vi "Main Comic Manager.vi"() -> ()   [LabVIEW 2024]
uses:
  <vilib>/sklein/WebView2/Webview2 Control/WebView2 Control.xctl
  definitions/volume.type--enum.ctl
  definitions/local_volume.ctl
  definitions/local_issue.ctl
  definitions/comicvine_issue.generic_credit.ctl
  definitions/comicvine_issue.associated_image.ctl
  definitions/comicvine_issue.person_credit.ctl
  <vilib>/addons/_JKI Toolkits/State Machine/_JKI_lib_State_Machine.llb/Select State(s)_err__jki_lib_state_machine.vi
  <vilib>/addons/_JKI Toolkits/State Machine/_JKI_lib_State_Machine.llb/Periodic Trigger__ogtk__JKI-SM__jki_lib_state_machine.vi
  <userlib>/_OpenG.lib/array/array.llb/Remove Duplicates from 1D Array (Variant)__ogtk.vi
  <userlib>/_OpenG.lib/file/file.llb/Strip Path Extension - String__ogtk.vi
  <userlib>/_OpenG.lib/file/file.llb/openg_file.lvlib
  <vilib>/addons/_JKI.lib/Serialization/JSON/JKI JSON Serialization.lvlib
  <userlib>/_OpenG.lib/array/array.llb/openg_array.lvlib
panel:
  in  "delete issue":bool caption="delete current"
  in  "use rel date":bool caption="delete current"
  out "issue chart":picture
  in  "fix dates":bool caption="delete current"
  out "dup issues":i32[](array[numeric])
  out "Unique Dates":bool
  in  "delete volume":bool caption="delete current"
  out "URL":string
  in  "refresh listings":bool
  in  "commit volume type":bool
  in  "volume type":T1 caption="Enum"
  out "last updated":string
  in  "Volume":i32 caption="Numeric"
  in  "issue detail tab control":enum32{"Details", "Cover", "Lists"}(tab)
  out "Rel Date":timestamp format="%<%x>T"
  out "Issue ID":i32 caption="Numeric"
  out "Issue Title":string
  in  "Cover Date":timestamp format="%<%x>T"
  out "Issue Number":string
  in  "issue description":string(xcontrol)
  in  "issue cover":string(xcontrol)
  out "Characters":string[](array[string])
  out "Teams":string[](array[string])
  out "StoryArcs":string[](array[string])
  out "Creators":string[](array[string])
  out "Concepts":string[](array[string])
  in  "sort volume":bool
  in  "to top":bool
  in  "move down":bool
  in  "move up":bool
  in  "issues":i32(listbox)
  out "Start Year":i32 caption="Numeric"
  out "issue count":i32 caption="Numeric"
  out "Sortable Title":string
  in  "Title":string
  in  "volume description":string(xcontrol)
  in  "volumes":i32(listbox)
  in  "Folder":i32(listbox)
  in  "Exit":bool
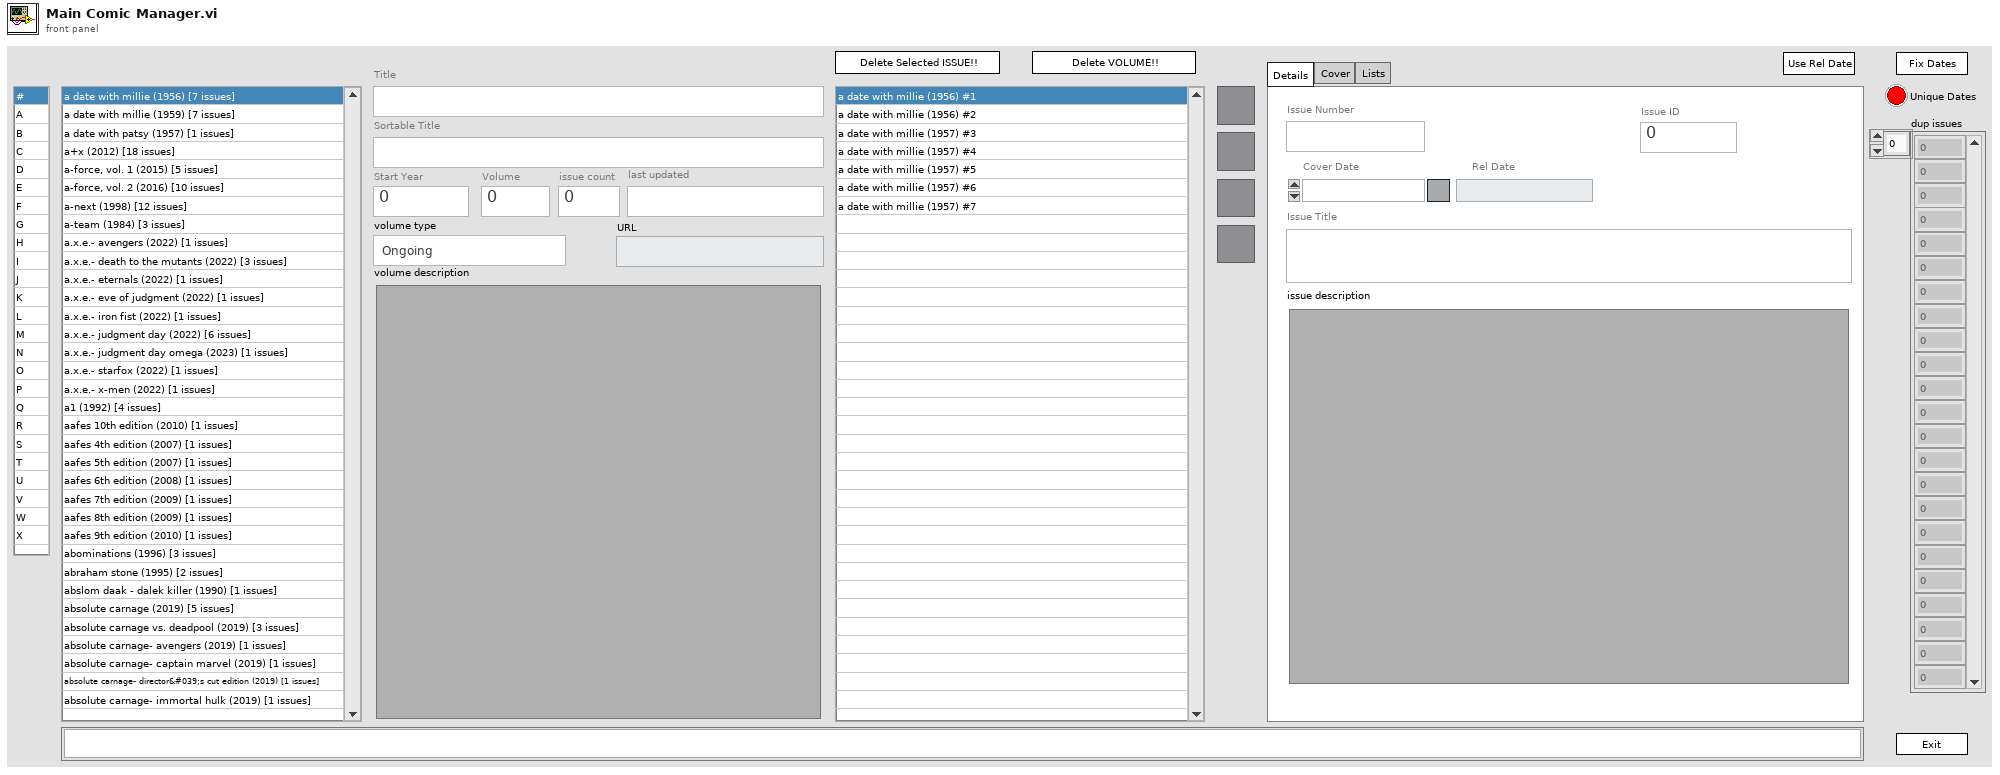
[diagram p1: front panel]
types:
  T1 = typedef "volume.type--enum.ctl" = enum16{"Ongoing", "Limited Series", "Annual", "One Shot", "Reprint/Document", "Star Comics", "Epic Comics"}
  T2 = enum32{"Invalid", "Standard", "Closed", "Hidden", "Minimized", "Maximized"}
  T3 = enum32{"invalid app kind", "Development System", "Run Time System", "Student Edition", "Embedded LabVIEW", "Evaluation", "Custom"}
  T4 = typedef "local_issue.ctl" = cluster{"cover_date":timestamp, "id":i32, "cv_id":string, "name":string, "sortable_name":string, "issue_number":string, "deck":string, "description":string, "volume":T5, "store_date":timestamp, "date_last_updated":timestamp, "site_detail_url":string, "cover_url":string, "associated_images":T6[], "characters":T5[], "concepts":T5[], "creators":T7[], "storyArcs":T5[], "teams":T5[]}
  T5 = typedef "comicvine_issue.generic_credit.ctl" = cluster{"id":i32, "name":string}
  T6 = typedef "comicvine_issue.associated_image.ctl" = cluster{"original_url":string, "id":i32}
  T7 = typedef "comicvine_issue.person_credit.ctl" = cluster{"id":i32, "name":string, "role":string}
  T8 = typedef "local_volume.ctl" = cluster{"id":i32, "name":string, "sortable_name":string, "aliases":string[], "description":string, "site_detail_url":string, "count_of_issues":i32, "start_year":i32, "publisher_id":i32, "issue_ids":i32[], "date_last_updated":timestamp, "volume":i32, "cv_id":string, "volume type":T1}
  T9 = cluster{"Core":cluster{"Current VI Reference":refnum<vi>, "Close Panel on Exit?":bool}, "cv_vols":path[], "vol_filter_map":map{i32, cluster{"name":string, "path":path}[]}, "current_vol_array":cluster{"name":string, "path":path}[], "volume":T8, "issues":T4[], "root paths":cluster{"cv_volumes":path, "cv_issues":path}, "dup issues":i32[]}
  T10 = cluster{"Current VI Reference":refnum<vi>, "Close Panel on Exit?":bool}
  T11 = typedef "WebView2 Control.xctl/Events.ctl" = cluster{"Navigation Complete Event":refnum<user-event>, "Source Changed Event":refnum<user-event>, "Document Title Changed Event":refnum<user-event>, "Status Bar Text Changed":refnum<user-event>, "Web Message Received":refnum<user-event>, "Window Close Requested":refnum<user-event>, "DOM Loaded":refnum<user-event>, "Navigation Started Event":refnum<user-event>}
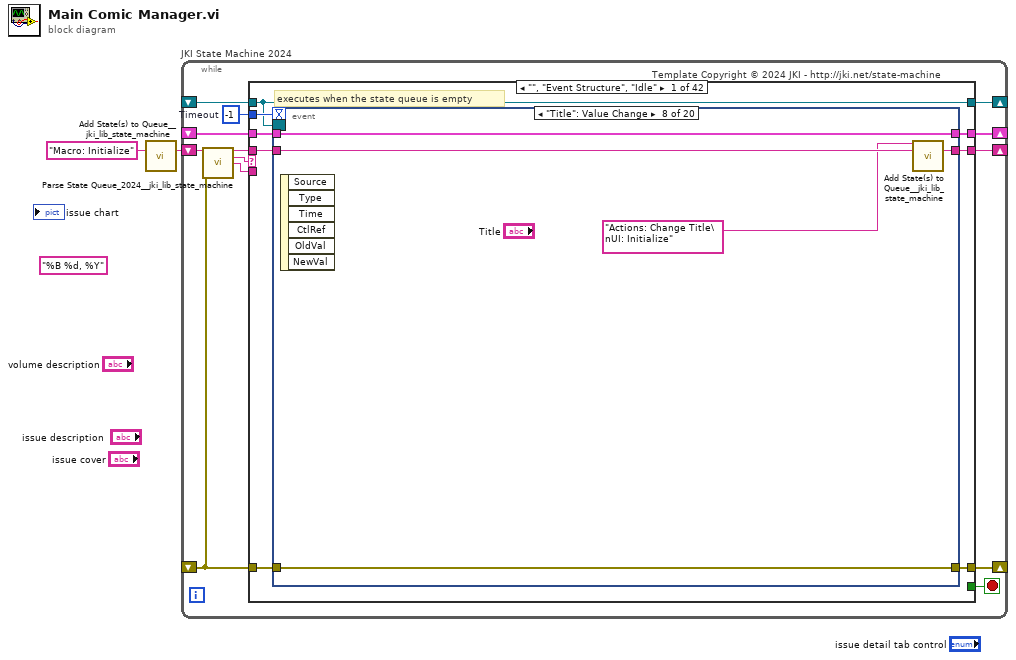
[diagram p0: block diagram]
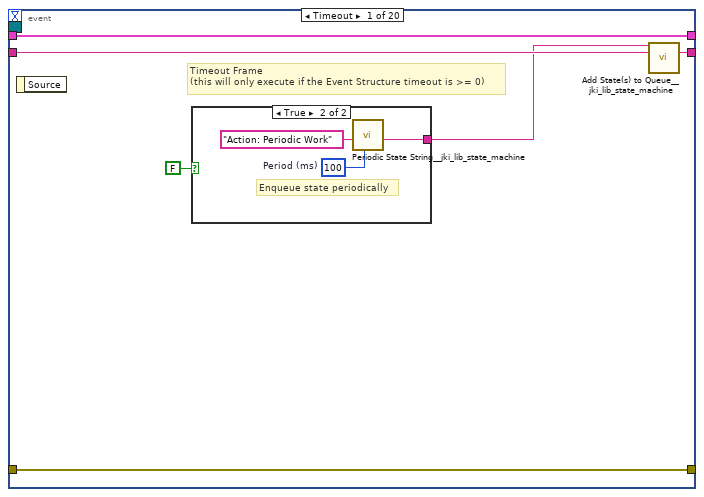
[diagram p2: hidden frame]
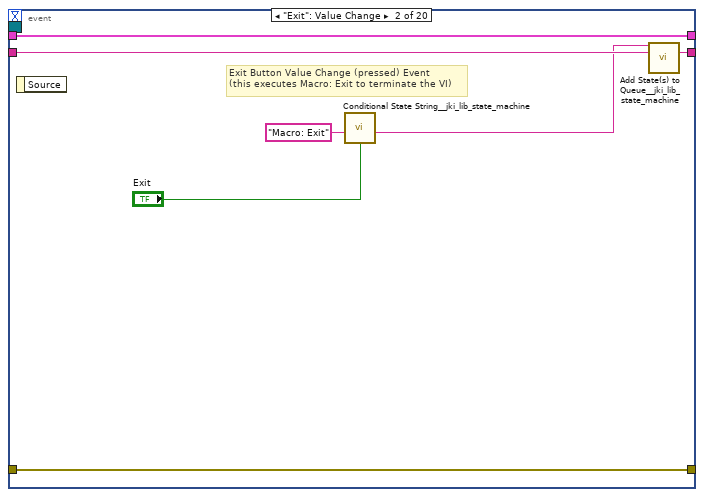
[diagram p4: hidden frame]
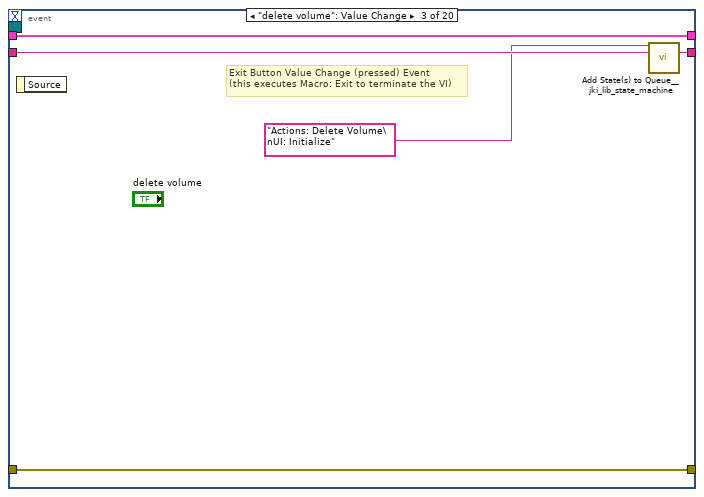
[diagram p5: hidden frame]
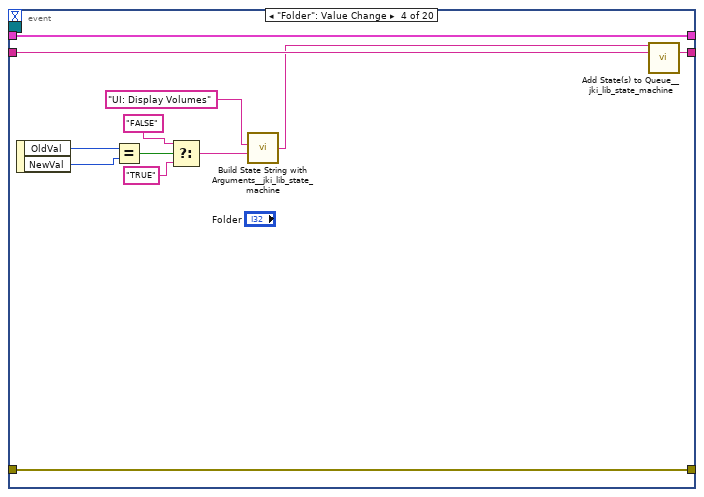
[diagram p6: hidden frame]
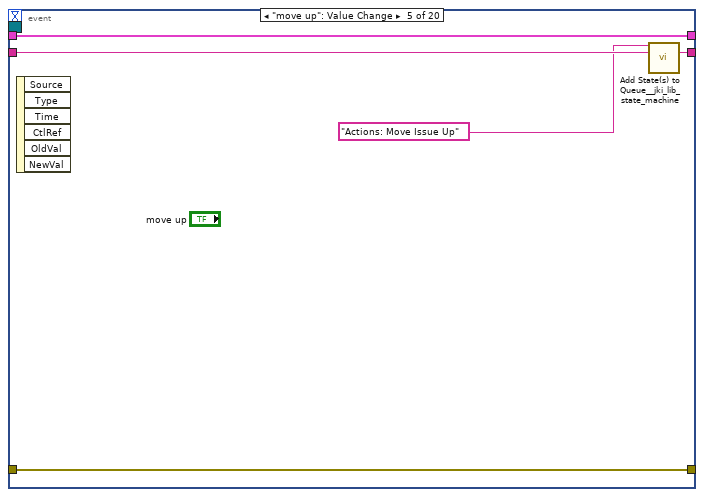
[diagram p7: hidden frame]
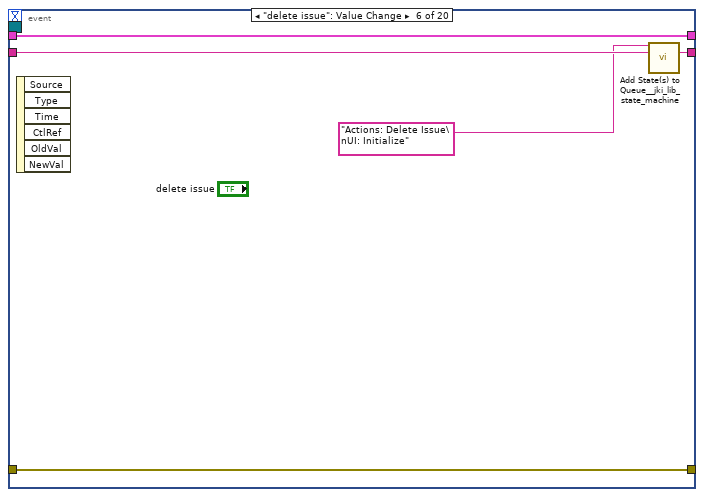
[diagram p8: hidden frame]
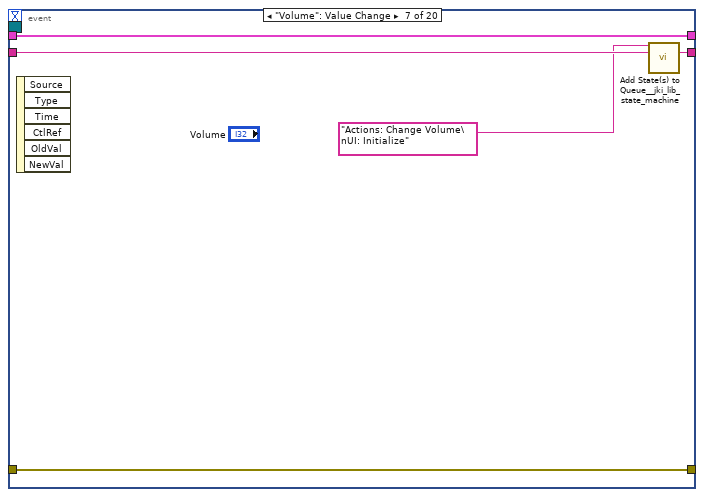
[diagram p9: hidden frame]
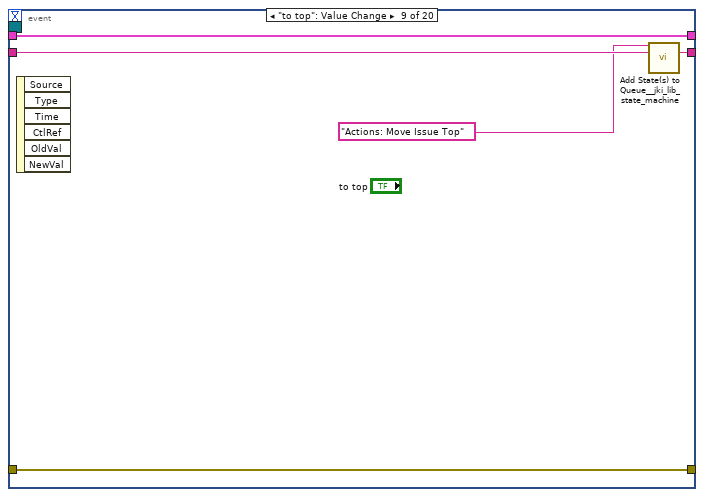
[diagram p10: hidden frame]
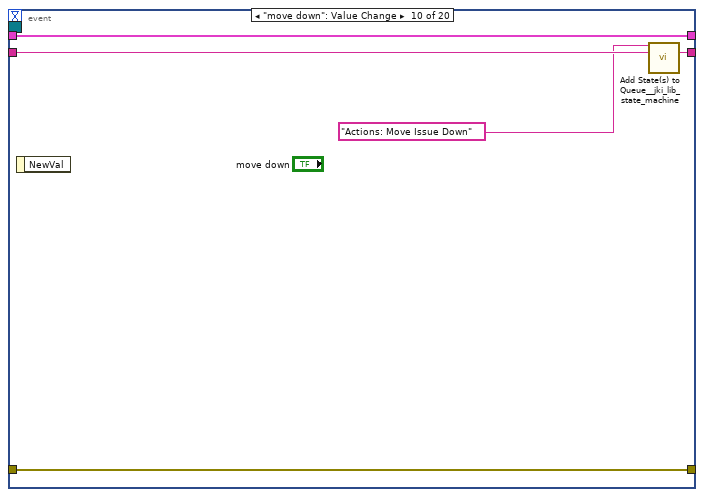
[diagram p11: hidden frame]
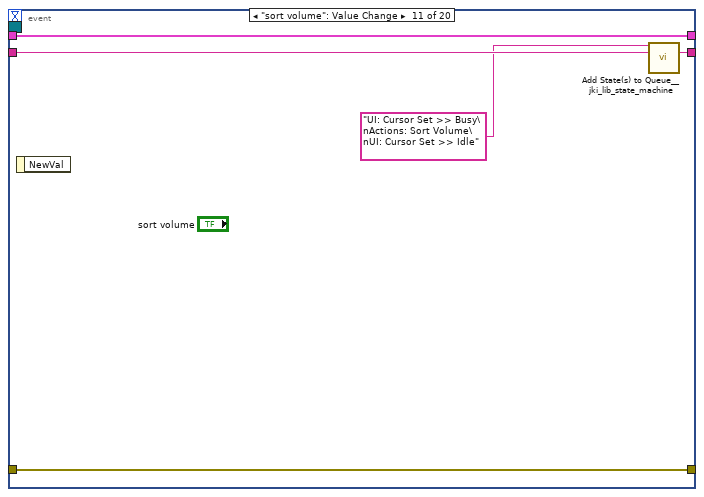
[diagram p12: hidden frame]
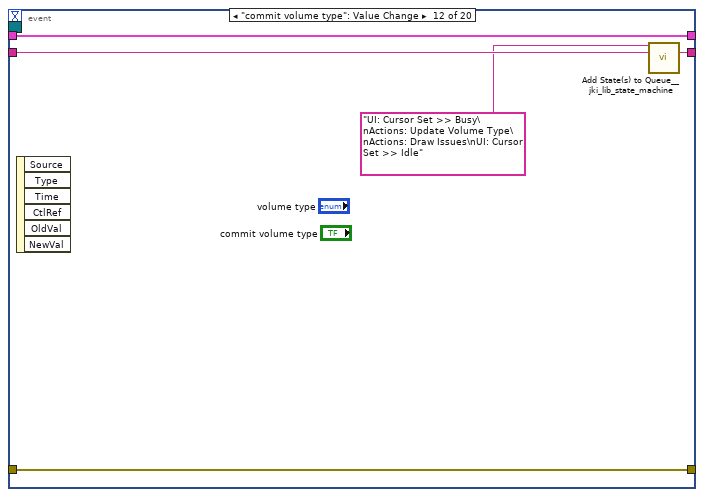
[diagram p13: hidden frame]
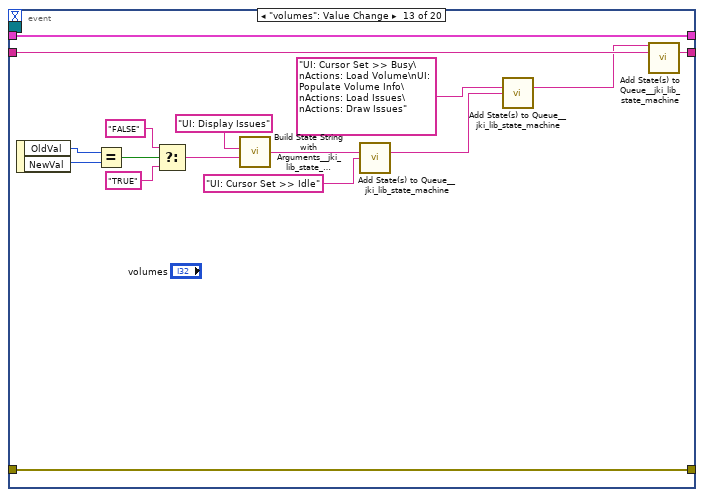
[diagram p14: hidden frame]
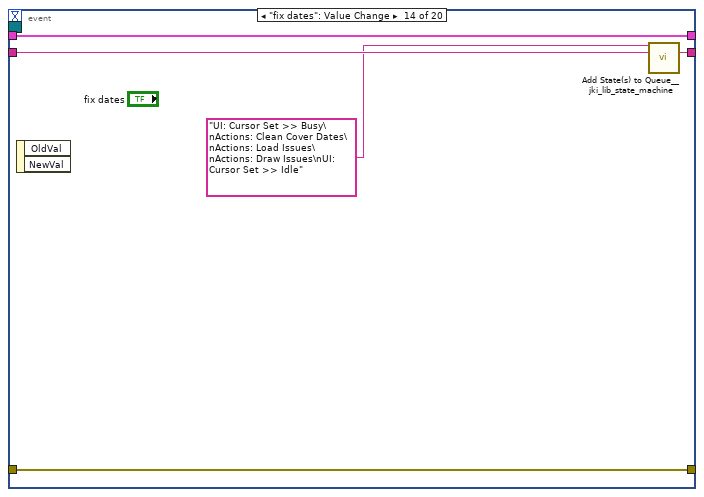
[diagram p15: hidden frame]
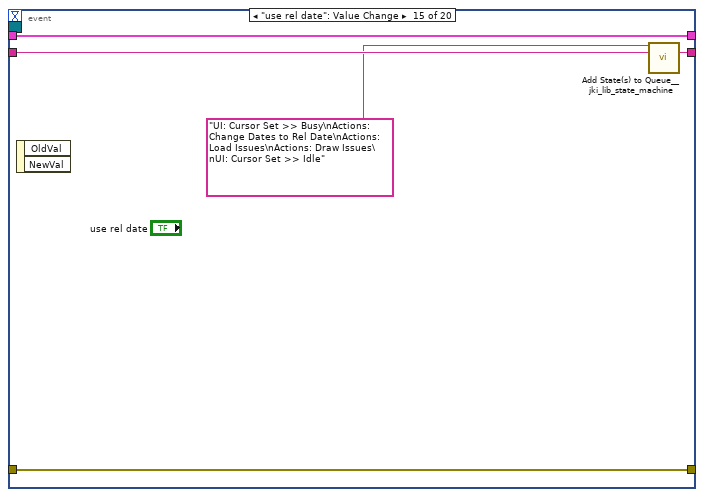
[diagram p16: hidden frame]
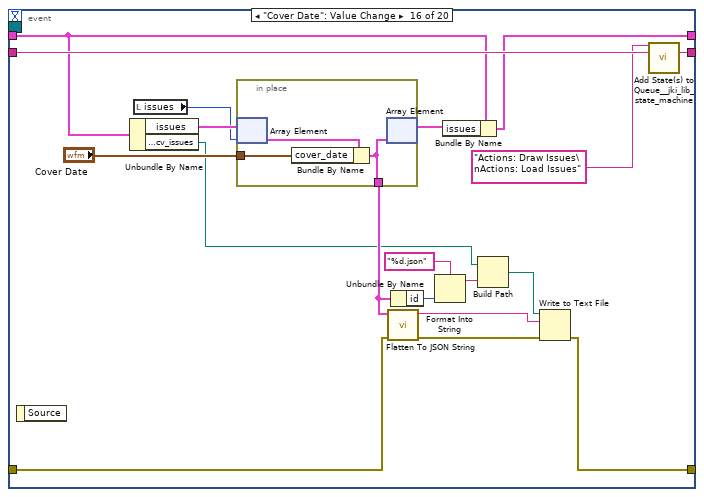
[diagram p17: hidden frame]
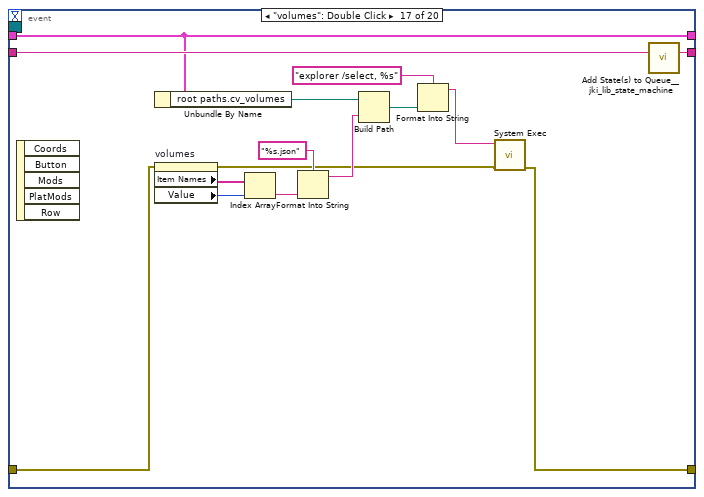
[diagram p18: hidden frame]
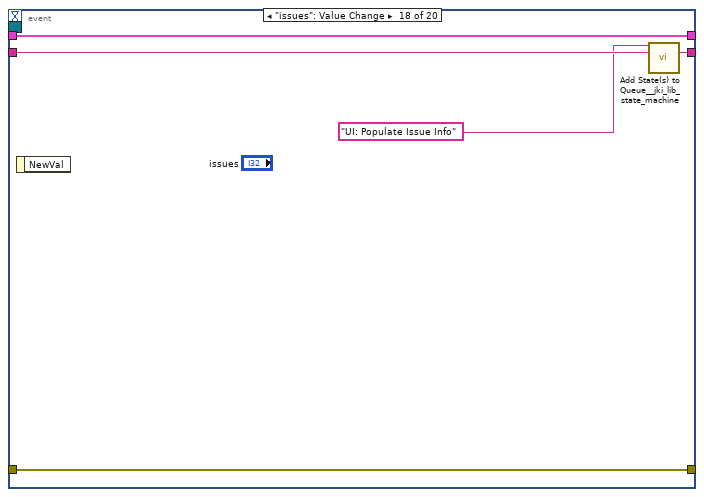
[diagram p19: hidden frame]
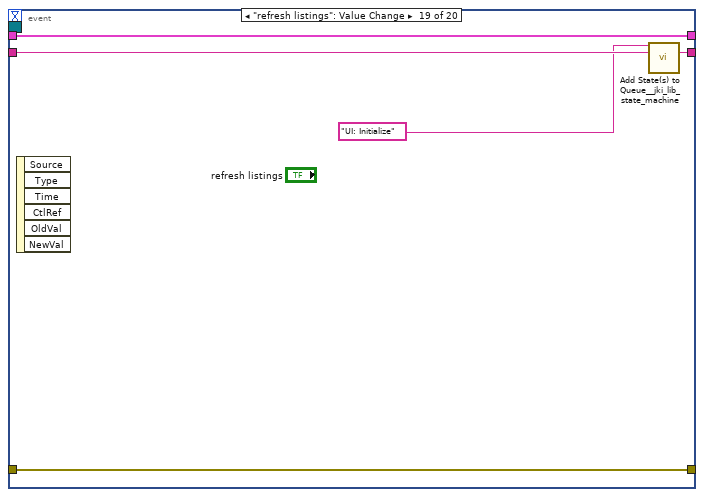
[diagram p20: hidden frame]
diagram:
  (unwired) "%B %d, %Y" ("time format string (%c)")
  n1 = call <vilib>:"Add State(s) to Queue__jki_lib_state_machine.vi"("State(s) in (\"\")"="Macro: Initialize") -> ("States Out"=w2:string)  [unwired: 14 in]
  n2 = while "JKI State Machine 2024" {
    shift-right: [w8] -> _
    shift-left: _ -> [w7]
    shift-right: [w11] -> _
    shift-left: _ -> [w5]
    shift-right: [w10] -> _
    shift-left: w2 -> [w12]
    shift-right: [w4] -> _
    shift-left: _ -> [w3]
    stop <- w9 stop-if-true
    w6 = -1  # Timeout
    # "Template Copyright © 2024 JKI - http://jki.net/state-machine"
    n3 = call <vilib>:"Parse State Queue_2024__jki_lib_state_machine.vi"("State Queue"=w12, "Error In (no error)"=w5) -> ("Remaining States"=w14:string, "Current State"=w15:string, "Arguments"=w13:string)  [unwired: 11 in]
    n4 = case shown="\"\", \"Event Structure\", \"Idle\"" w15 {
      selector: w15 -> [_ _ w182 _ _ _ _ _ _ _ _ _ _ _ _ _ _ _ _ _ _ _ _ _ _ _ _ _ _ _ _ _ _ _ _ _ _ _ _ _ _ _]
      tunnel: w14 -> [w23 w180 w186 w206 w217 w227 w232 w245 w252 w257 w267 w273 w278 w291 w310 w331 w347 w376 w395 w400 w407 w419 w489 w495 w505 w510 w536 w556 w581 w591 w616 w630 w655 w674 w691 w713 w737 w759 w776 w789 w825 w836]
      tunnel: w13 -> [_ _ _ _ w212 _ _ _ _ _ _ _ _ w279 w302 _ _ _ _ _ w402 w413 _ _ _ _ _ _ _ _ _ _ _ _ _ _ _ _ _ _ _ _]
      tunnel: w7 -> [w21 w177 w184 w199 w214 w225 w229 _ w247 w254 w265 w271 w275 w287 w305 w328 w342 w373 w393 w398 w405 w415 w486 w492 w503 w507 w527 w551 w576 w586 w613 w625 w652 w670 w677 w710 w734 w756 w762 w784 w817 w831]
      tunnel: [w20 w178 w188 w203 errorcluster {"status"=FALSE, "code"=0, "source"=""} ("error out") w224 w230 w242 w248 w255 w259 w268 w276 w282 w306 w329 w344 w362 w392 w397 w403 w416 w487 w493 w500 w508 w513 w538 w563 w583 w607 w620 w643 w666 w679 w693 w716 w739 w764 w781 w820 w828] -> w11
      tunnel: w5 -> [w17 w178 w187 w203 w213 w224 w230 w242 w249 w255 w261 w269 w276 w283 w307 w329 w345 w365 w392 w397 w404 w417 w487 w493 w500 w508 w522 w546 w571 w582 w608 w621 w645 w671 w685 w700 w724 w746 w770 w785 w819 w827]
      tunnel: [w22 w179 w185 w205 w216 w226 w231 w244 w251 w256 w266 w272 w277 w290 w309 w330 w346 w375 w394 w399 w406 w418 w488 w494 w504 w509 w535 w555 w580 w590 w615 w629 w654 w673 w690 w712 w736 w758 w775 w789 w824 w836] -> w10
      tunnel: [_ _ _ _ _ TRUE _ _ _ _ _ _ _ _ _ _ _ _ _ _ _ _ _ _ _ _ _ _ _ _ _ _ _ _ _ _ _ _ _ _ _ _] -> w9
      tunnel: [w19 w177 w184 w204 w214 w225 w229 w243 w247 w254 w265 w271 w275 w286 w305 w328 w342 w373 w393 w398 w405 w415 w486 w492 w503 w507 w531 w553 w578 w584 w613 w624 w652 w670 w675 w710 w734 w756 w761 w782 w821 w829] -> w8
      tunnel: w6 -> [w18 _ _ _ _ _ _ _ _ _ _ _ _ _ _ _ _ _ _ _ _ _ _ _ _ _ _ _ _ _ _ _ _ _ _ _ _ _ _ _ _ _]
      tunnel: [w16 w176 w181 w193 w207 w222 w228 w237 w246 w253 w262 w270 w274 w281 w308 w327 w343 w374 w390 w396 w401 w412 w485 w490 w496 w506 w534 w554 w579 w589 w614 w628 w653 w672 w689 w711 w735 w757 w763 w788 w818 w826] -> w4
      tunnel: w3 -> [w16 w176 w181 w193 w207 w222 w228 w237 w246 w253 _ w270 w274 w281 w308 w327 w343 w374 w390 w396 w401 w412 w485 w490 w496 w506 w534 w554 w579 w589 w614 w628 w653 w672 w689 w711 w735 w757 w763 w788 w818 w826]
      frame "", "Event Structure", "Idle" {
        # "executes when the state queue is empty"
        n5 = event shown="[7] \"Title\": Value Change" {
          selector: w16 -> [_ _ _ _ _ _ _ _ _ _ _ _ _ _ _ _ _ _ _ _]
          dyn-events: _ -> [_ _ _ _ _ _ _ _ _ _ _ _ _ _ _ _ _ _ _ _]
          timeout: w18 -> [_ _ _ _ _ _ _ _ _ _ _ _ _ _ _ _ _ _ _ _]
          tunnel: w23 -> [w29 w39 w44 w56 w61 w66 w71 w76 w81 w86 w91 w96 w112 w117 w122 w141 w159 w164 w169 w175]
          tunnel: [w28 w38 w43 w55 w60 w65 w70 w75 w80 w85 w90 w95 w111 w116 w121 w140 w158 w163 w168 w174] -> w22
          tunnel: w21 -> [w26 w36 w41 w53 w58 w63 w68 w73 w78 w83 w88 w93 w109 w114 w119 w136 w153 w161 w166 w172]
          tunnel: [w27 w37 w42 w54 w59 w64 w69 w74 w79 w84 w89 w94 w110 w115 w120 w124 w145 w162 w167 w173] -> w20
          tunnel: w17 -> [w27 w37 w42 w54 w59 w64 w69 w74 w79 w84 w89 w94 w110 w115 w120 w133 w150 w162 w167 w173]
          tunnel: [w26 w36 w41 w53 w58 w63 w68 w73 w78 w83 w88 w93 w109 w114 w119 w134 w153 w161 w166 w172] -> w19
          event Timeout {
            # "Timeout Frame\n(this will only execute if the Event Structure timeout is >= 0)"
            n6 = event-data() -> ()  [unwired: 1 in, 1 out]
            n7 = case shown="True" FALSE {
              tunnel: [_ w32] -> w25
              frame False {
              }
              frame True {
                w30 = u32 100  # Period (ms)
                # "Enqueue state periodically"
                n8 = call <vilib>:"Periodic State String__jki_lib_state_machine.vi"("Period (ms)"=w30, "State"="Action: Periodic Work") -> ("State Out"=w32:string)  [unwired: 9 in]
              }
            }
            n9 = call <vilib>:"Add State(s) to Queue__jki_lib_state_machine.vi"("State(s) in Front (\"\")"=w25, "State(s) in (\"\")"=w29) -> ("States Out"=w28:string)  [unwired: 13 in]
          }
          event "Exit": Value Change {
            # "Exit Button Value Change (pressed) Event\n(this executes Macro: Exit to terminate the VI)"
            n10 = event-data() -> ()  [unwired: 1 in, 1 out]
            n11 = call <vilib>:"Conditional State String__jki_lib_state_machine.vi"("Do State(s)?"="Exit", "State"="Macro: Exit") -> ("State Out"=w33:string)  [unwired: 7 in]
            n12 = call <vilib>:"Add State(s) to Queue__jki_lib_state_machine.vi"("State(s) in Front (\"\")"=w33, "State(s) in (\"\")"=w39) -> ("States Out"=w38:string)  [unwired: 13 in]
          }
          event "delete volume": Value Change {
            # "Exit Button Value Change (pressed) Event\n(this executes Macro: Exit to terminate the VI)"
            n13 = event-data() -> ()  [unwired: 1 in, 1 out]
            n14 = call <vilib>:"Add State(s) to Queue__jki_lib_state_machine.vi"("State(s) in Front (\"\")"="Actions: Delete Volume\nUI: Initialize", "State(s) in (\"\")"=w44) -> ("States Out"=w43:string)  [unwired: 13 in]
          }
          event "Folder": Value Change {
            n15 = event-data() -> ("OldVal"=w52:i32, "NewVal"=w51:i32)  [unwired: 1 in]
            n16 = Equal?(x=w52, y=w51) -> (x = y?=w50:bool)
            n17 = Select(t="FALSE", s=w50, f="TRUE") -> (s? t:f=w46:string)
            n18 = call <vilib>:"Build State String with Arguments__jki_lib_state_machine.vi"("Arguments (\"\")"=w46, "State"="UI: Display Volumes") -> ("State with Arguments"=w45:string)  [unwired: 4 in]
            n19 = call <vilib>:"Add State(s) to Queue__jki_lib_state_machine.vi"("State(s) in Front (\"\")"=w45, "State(s) in (\"\")"=w56) -> ("States Out"=w55:string)  [unwired: 13 in]
          }
          event "move up": Value Change {
            n20 = event-data() -> ()  [unwired: 1 in, 6 out]
            n21 = call <vilib>:"Add State(s) to Queue__jki_lib_state_machine.vi"("State(s) in Front (\"\")"="Actions: Move Issue Up", "State(s) in (\"\")"=w61) -> ("States Out"=w60:string)  [unwired: 13 in]
          }
          event "delete issue": Value Change {
            n22 = event-data() -> ()  [unwired: 1 in, 6 out]
            n23 = call <vilib>:"Add State(s) to Queue__jki_lib_state_machine.vi"("State(s) in Front (\"\")"="Actions: Delete Issue\nUI: Initialize", "State(s) in (\"\")"=w66) -> ("States Out"=w65:string)  [unwired: 13 in]
          }
          event "Volume": Value Change {
            n24 = event-data() -> ()  [unwired: 1 in, 6 out]
            n25 = call <vilib>:"Add State(s) to Queue__jki_lib_state_machine.vi"("State(s) in Front (\"\")"="Actions: Change Volume\nUI: Initialize", "State(s) in (\"\")"=w71) -> ("States Out"=w70:string)  [unwired: 13 in]
          }
          event "Title": Value Change {
            n26 = event-data() -> ()  [unwired: 1 in, 6 out]
            n27 = call <vilib>:"Add State(s) to Queue__jki_lib_state_machine.vi"("State(s) in Front (\"\")"="Actions: Change Title\nUI: Initialize", "State(s) in (\"\")"=w76) -> ("States Out"=w75:string)  [unwired: 13 in]
          }
          event "to top": Value Change {
            n28 = event-data() -> ()  [unwired: 1 in, 6 out]
            n29 = call <vilib>:"Add State(s) to Queue__jki_lib_state_machine.vi"("State(s) in Front (\"\")"="Actions: Move Issue Top", "State(s) in (\"\")"=w81) -> ("States Out"=w80:string)  [unwired: 13 in]
          }
          event "move down": Value Change {
            n30 = event-data() -> ()  [unwired: 1 in, 1 out]
            n31 = call <vilib>:"Add State(s) to Queue__jki_lib_state_machine.vi"("State(s) in Front (\"\")"="Actions: Move Issue Down", "State(s) in (\"\")"=w86) -> ("States Out"=w85:string)  [unwired: 13 in]
          }
          event "sort volume": Value Change {
            n32 = event-data() -> ()  [unwired: 1 in, 1 out]
            n33 = call <vilib>:"Add State(s) to Queue__jki_lib_state_machine.vi"("State(s) in Front (\"\")"="UI: Cursor Set >> Busy\nActions: Sort Volume\nUI: Cursor Set >> Idle", "State(s) in (\"\")"=w91) -> ("States Out"=w90:string)  [unwired: 13 in]
          }
          event "commit volume type": Value Change {
            n34 = event-data() -> ()  [unwired: 1 in, 6 out]
            n35 = call <vilib>:"Add State(s) to Queue__jki_lib_state_machine.vi"("State(s) in Front (\"\")"="UI: Cursor Set >> Busy\nActions: Update Volume Type\nActions: Draw Issues\nUI: Cursor Set >> Idle", "State(s) in (\"\")"=w96) -> ("States Out"=w95:string)  [unwired: 13 in]
          }
          event "volumes": Value Change {
            n36 = event-data() -> ("OldVal"=w107:i32, "NewVal"=w108:i32)  [unwired: 1 in]
            n37 = Equal?(x=w107, y=w108) -> (x = y?=w104:bool)
            n38 = Select(t="FALSE", s=w104, f="TRUE") -> (s? t:f=w102:string)
            n39 = call <vilib>:"Build State String with Arguments__jki_lib_state_machine.vi"("Arguments (\"\")"=w102, "State"="UI: Display Issues") -> ("State with Arguments"=w99:string)  [unwired: 4 in]
            n40 = call <vilib>:"Add State(s) to Queue__jki_lib_state_machine.vi"("State(s) in (\"\")"=w99, "State(s) at Back (\"\")"="UI: Cursor Set >> Idle" ("State(s) at Back (\"\")")) -> ("States Out"=w98:string)  [unwired: 13 in]
            n41 = call <vilib>:"Add State(s) to Queue__jki_lib_state_machine.vi"("State(s) in (\"\")"="UI: Cursor Set >> Busy\nActions: Load Volume\nUI: Populate Volume Info\nActions: Load Issues\nActions: Draw Issues", "State(s) at Back (\"\")"=w98) -> ("States Out"=w105:string)  [unwired: 13 in]
            n42 = call <vilib>:"Add State(s) to Queue__jki_lib_state_machine.vi"("State(s) in Front (\"\")"=w105, "State(s) in (\"\")"=w112) -> ("States Out"=w111:string)  [unwired: 13 in]
          }
          event "fix dates": Value Change {
            n43 = event-data() -> ()  [unwired: 1 in, 2 out]
            n44 = call <vilib>:"Add State(s) to Queue__jki_lib_state_machine.vi"("State(s) in Front (\"\")"="UI: Cursor Set >> Busy\nActions: Clean Cover Dates\nActions: Load Issues\nActions: Draw Issues\nUI: Cursor Set >> Idle", "State(s) in (\"\")"=w117) -> ("States Out"=w116:string)  [unwired: 13 in]
          }
          event "use rel date": Value Change {
            n45 = event-data() -> ()  [unwired: 1 in, 2 out]
            n46 = call <vilib>:"Add State(s) to Queue__jki_lib_state_machine.vi"("State(s) in Front (\"\")"="UI: Cursor Set >> Busy\nActions: Change Dates to Rel Date\nActions: Load Issues\nActions: Draw Issues\nUI: Cursor Set >> Idle", "State(s) in (\"\")"=w122) -> ("States Out"=w121:string)  [unwired: 13 in]
          }
          event "Cover Date": Value Change {
            n47 = event-data() -> ()  [unwired: 1 in, 1 out]
            n48 = Unbundle By Name(w136) -> ("issues"=w138:T4[], "root paths.cv_issues"=w128:path)
            n49 = local read "issues"() -> (w137:i32)
            n50 = in-place {
              in-place-border: "Cover Date" -> [w143]
              in-place-border: [w142] -> w132
              n51 = in-place-array #1(w138, w137) -> (w144:T4)
              n52 = Bundle By Name(cluster=w144, "cover_date"=w143) -> (w142:T4)
              n53 = in-place-array #1(w142) -> (w135:T4[])  [unwired: 1 out]
            }
            n54 = call <vilib>:"Flatten To JSON String.vi"("error in"=w133, "Variant"=w132) -> ("error out"=w125:errorcluster, "JSON String"=w126:string)  [unwired: 8 in]
            n55 = Unbundle By Name(w132) -> ("id"=w131:i32)
            n56 = Format Into String(format string="%d.json", w131) -> (resulting string=w129:string)  [unwired: 2 in, 1 out]
            n57 = Bundle By Name(cluster=w136, "issues"=w135) -> (w134:T9)
            n58 = Build Path(base path=w128, name or relative path=w129) -> (appended path=w127:path)
            n59 = Write to Text File(file (use dialog)=w127, text=w126, error in=w125) -> (error out=w124:errorcluster)  [unwired: 1 in, 2 out]
            n60 = call <vilib>:"Add State(s) to Queue__jki_lib_state_machine.vi"("State(s) in Front (\"\")"="Actions: Draw Issues\nActions: Load Issues" ("State(s) in Front (\"\")"), "State(s) in (\"\")"=w141) -> ("States Out"=w140:string)  [unwired: 13 in]
          }
          event "volumes": Double Click {
            n61 = event-data() -> ()  [unwired: 1 in, 5 out]
            n62 = Unbundle By Name(w153) -> ("root paths.cv_volumes"=w152:path)
            n63 = property on="volumes" class="LstBox (strict)"(error in=w150) -> (error out=w146:errorcluster, "Item Names"=w156:string[], "Value"=w157:i32)  [unwired: 1 in, 1 out]
            n64 = Index Array(array=w156, index=w157) -> (element=w154:string)
            n65 = Format Into String(format string="%s.json", w154) -> (resulting string=w151:string)  [unwired: 2 in, 1 out]
            n66 = Build Path(base path=w152, name or relative path=w151) -> (appended path=w148:path)
            n67 = Format Into String(format string="explorer /select, %s", w148) -> (resulting string=w147:string)  [unwired: 2 in, 1 out]
            n68 = call <vilib>:"System Exec.vi"("error in (no error)"=w146, "command line"=w147) -> ("error out"=w145:errorcluster)  [unwired: 6 in, 3 out]
            n69 = call <vilib>:"Add State(s) to Queue__jki_lib_state_machine.vi"("State(s) in (\"\")"=w159) -> ("States Out"=w158:string)  [unwired: 14 in]
          }
          event "issues": Value Change {
            n70 = event-data() -> ()  [unwired: 1 in, 1 out]
            n71 = call <vilib>:"Add State(s) to Queue__jki_lib_state_machine.vi"("State(s) in Front (\"\")"="UI: Populate Issue Info", "State(s) in (\"\")"=w164) -> ("States Out"=w163:string)  [unwired: 13 in]
          }
          event "refresh listings": Value Change {
            n72 = event-data() -> ()  [unwired: 1 in, 6 out]
            n73 = call <vilib>:"Add State(s) to Queue__jki_lib_state_machine.vi"("State(s) in Front (\"\")"="UI: Initialize", "State(s) in (\"\")"=w169) -> ("States Out"=w168:string)  [unwired: 13 in]
          }
          event Panel Close? {
            # "Discard the event because we'll close the front panel ourselves in Macro: Exit"
            # "Close Panel button (pressed) Event\n(this executes Macro: Exit to terminate the VI)"
            n74 = event-data() -> ()  [unwired: 1 in, 1 out]
            n75 = event-data("Discard?"=TRUE) -> ()  [unwired: 1 in, 1 out]
            n76 = call <vilib>:"Add State(s) to Queue__jki_lib_state_machine.vi"("State(s) in Front (\"\")"="Macro: Exit", "State(s) in (\"\")"=w175) -> ("States Out"=w174:string)  [unwired: 13 in]
          }
        }
      }
      frame "---------- Core ----------" {
        # "Do not put any code in this frame.\n(it is a separator no-op)"
        n77 = call <vilib>:"Add State(s) to Queue__jki_lib_state_machine.vi"("State(s) in (\"\")"=w180) -> ("States Out"=w179:string)  [unwired: 14 in]
      }
      frame Default {
        w191 = 42 items=["No error", "Argument error", "Memory is full", "Out of zone", "End of file", "File already open", "Generic file I/O error", "File not found", "File permission error", "Disk is full", "Duplicate path", "Too many files open", "System feature not enabled", "Resource file not found", "Cannot add resource", "Resource not found", "Image not found", "Image memory error", "Pen does not exist", "Config type invalid", "Config token not found", "Config parse error", "Config memory error", "Bad external code format", "Bad external code offset", "External code not present", "Null window", "Destroy window error", "Null menu", "Print aborted", "Bad print record", "Print driver error", "Windows error during printing", "Memory error during printing", "Print dialog error", "Generic print error", "Invalid device refnum", "Device not found", "Device parameter error", "Device unit error", "Cannot open device", "Device call aborted", "Generic error", "Cancelled by user", "Object ID too low", "Object ID too high", "Object not in heap", "Unknown heap", "Unknown object (invalid DefProc)", "Unknown object (DefProc not in table)", "Message out of range", "Invalid (null) method", "Unknown message", "Manager call not supported", "Bad address", "Network operation in progress", "Network operation timed out", "Connection is busy", "Network attribute not supported", "Network error", "Address in use", "System out of memory", "Connection aborted", "Connection refused", "Not connected", "Already connected", "Connection closed", "Initialization error (interapplication manager)", "Bad occurrence", "Wait on unbound occurrence handler", "Occurrence queue overflow", "Datalog type conflict", "Unused", "Unrecognized type (interapplication manager)", "Memory corrupt", "Failed to make temporary DLL", "Old CIN version", "Drag socket not found", "Failed to load drop-object", "Failed to register OLE object", "Failed to release OLE object", "Format specifier type mismatch", "Unknown format specifier", "Too few format specifiers", "Too many format specifiers", "Scan failed", "Newer CIN version", "Error converting to variant", "Runtime menu error", "Password tampered", "Variant attribute not found", "Incompatible variant data type", "Event data is not available", "Event Store is not present", "Occurrence is not found", "Event Queue is not created", "Event info is not available", "Refnum passed is NULL", "Error retrieving Class GUID", "Error retrieving CoClass GUID", "Error retrieving TypeLib GUID.", "Bad built application magic bytes.", "Specific driver is different from the specific driver associated with the Logical Name.", "There is no session opened to the class driver.", "Max Error", "MAX - Error with config objects", "MAX - Error loading configuration", "MAX - Group not supported"]
        # "Current State"
        # "Do not delete, rename, or modify this frame.\n(this is used to capture unhandled states and typos)"
        # "Handle mistyped state name (developer tool)"
        n78 = Format Into String(format string="Software Exception: Unhandled State \"%s\"." ("message"), error in=w187, w182) -> (resulting string=w190:string, error out=w189:errorcluster)  [unwired: 1 in]
        n79 = call <vilib>:"Error Cluster From Error Code.vi"("show call chain? (False)"=TRUE, "error in (no error)"=w189, "error message (\"\")"=w190, "error code (0)"=w191) -> ("error out"=w188:errorcluster)  [unwired: 5 in]
        n80 = call <vilib>:"Add State(s) to Queue__jki_lib_state_machine.vi"("State(s) in (\"\")"=w186) -> ("States Out"=w185:string)  [unwired: 14 in]
      }
      frame "Initialize Core Data" {
        # "Do not delete, rename, or modify this frame.\n(this is used to determine panel behavior on exit)"
        # "originally closed?"
        # "exe?"
        # "If panel starts closed or is an EXE, then close it when we exit"
        n81 = property class="VI"() -> ("FP.State"=w196:T2)  [unwired: 2 in, 2 out]
        n82 = property class="App"() -> ("App.Kind"=w202:T3)  [unwired: 2 in, 2 out]
        n83 = control-ref of="Current VI Reference"() -> (w197:refnum<vi>)
        n84 = Equal?(x=w196, y=T2."Closed" ("Front Panel Window:State")) -> (x = y?=w194:bool)
        n85 = Equal?(x=w202, y=T3."Run Time System" ("Application:Kind")) -> (x = y?=w200:bool)
        n86 = Or(x=w194, y=w200) -> (x .or. y?=w198:bool)
        n87 = Bundle By Name(cluster=w199, "Core.Current VI Reference"=w197, "Core.Close Panel on Exit?"=w198) -> (w204:T9)
        n88 = call <vilib>:"Add State(s) to Queue__jki_lib_state_machine.vi"("State(s) in (\"\")"=w206) -> ("States Out"=w205:string)  [unwired: 14 in]
      }
      frame "Error Handler" {
        # "When running as sourcecode, this function will add previous state data to the error message to aid the developer in troubleshoot errors.\nIf run as an executable, no additional information is added to the error message."
        # "This state receives both Errors and Warnings which is how the Status of this wire can be FALSE"
        # "Unhandled Error -- Display it"
        # "Handle any errors or warnings here.\nYou can also output any states to clean-up after errors or warnings occur"
        # "Clear error or warning"
        n89 = disable-structure shown="Default" {
          disable-tunnel: w213 -> [w220 w221]
          disable-tunnel: w212 -> [w219 _]
          disable-tunnel: [w218 w221] -> w211
          frame condition #0 (active) {
            n90 = call <vilib>:"Append Error Details__jki_lib_state_machine.vi"("error in (no error)"=w220, "Previous State and Argument(s)"=w219) -> ("error out"=w218:errorcluster)  [unwired: 9 in]
          }
          frame condition #1 {
          }
        }
        n91 = call <vilib>:"General Error Handler.vi"("error in (no error)"=w211) -> ()  [unwired: 10 in, 5 out]
        n92 = call-poly <vilib>:"Select State(s)__jki_lib_state_machine.vi"("State(s) if True (\"\")"="/* Post Error States", "Select"=w211, "State(s) if False (\"\")"="/* Post Warning States") -> ("States Out"=w209:string)  [unwired: 12 in]
        n93 = call <vilib>:"Add State(s) to Queue__jki_lib_state_machine.vi"("State(s) in Front (\"\")"=w209, "State(s) in (\"\")"=w217) -> ("States Out"=w216:string)  [unwired: 13 in]
      }
      frame "Exit" {
        # "Do not put any code in this frame.\n(No errors that occur here will be handled.)"
        n94 = call <vilib>:"Add State(s) to Queue__jki_lib_state_machine.vi"("State(s) in (\"\")"=w227) -> ("States Out"=w226:string)  [unwired: 14 in]
      }
      frame "---------- Data ----------" {
        # "Do not put any code in this frame.\n(It is a separator no-op. You can make a copy of this frame to create a new Data frame)"
        n95 = call <vilib>:"Add State(s) to Queue__jki_lib_state_machine.vi"("State(s) in (\"\")"=w232) -> ("States Out"=w231:string)  [unwired: 14 in]
      }
      frame "Data: Initialize" {
        w233 = i32[] []  # dup issues
        w234 = cluster{"cv_volumes":path, "cv_issues":path} {"cv_volumes"=path "D:/Comics/data/cv_volumes", "cv_issues"=path "D:/Comics/data/cv_issues"}  # root paths
        w235 = T4[] []  # issues
        w236 = T8 {"id"=0, "name"="", "sortable_name"="", "aliases"=[], "description"="", "site_detail_url"="", "count_of_issues"=0, "start_year"=0, "publisher_id"=0, "issue_ids"=[], "date_last_updated"=timestamp(0 s since 1904-01-01), "volume"=0, "cv_id"="", "volume type"=enum."One Shot"}  # volume
        w238 = cluster{"name":string, "path":path}[] []  # current_vol_array
        w239 = map{i32, cluster{"name":string, "path":path}[]} {}  # vol_filter_map
        w240 = path[] []  # cv_vols
        w241 = T10 {"Current VI Reference"=refnum, "Close Panel on Exit?"=FALSE}  # Core
        # "Data names and types of shift register data are defined by this bundle."
        # "Initialize the shift-register data, here.\n(data names are defined by what you wire into the bundle function)"
        n96 = Bundle("Core"=w241, "cv_vols"=w240, "vol_filter_map"=w239, "current_vol_array"=w238, "volume"=w236, "issues"=w235, "root paths"=w234, "dup issues"=w233) -> (w243:T9)  [unwired: 1 in]
        n97 = call <vilib>:"Add State(s) to Queue__jki_lib_state_machine.vi"("State(s) in (\"\")"=w245) -> ("States Out"=w244:string)  [unwired: 14 in]
      }
      frame "Data: Cleanup" {
        # "Cleanup any data and references, here.\n(this is called automatically, by the Macro: Exit)"
        n98 = Unbundle By Name(w247) -> ("Core.Current VI Reference"=w250:refnum<vi>)
        n99 = Close Reference(reference=w250, error in (no error)=w249) -> (error out=w248:errorcluster)
        n100 = call <vilib>:"Add State(s) to Queue__jki_lib_state_machine.vi"("State(s) in (\"\")"=w252) -> ("States Out"=w251:string)  [unwired: 14 in]
      }
      frame "---------- Events ----------" {
        n101 = call <vilib>:"Add State(s) to Queue__jki_lib_state_machine.vi"("State(s) in (\"\")"=w257) -> ("States Out"=w256:string)  [unwired: 14 in]
      }
      frame "Events: Register" {
        w263 = cluster{"My Event Data":bool} {"My Event Data"=FALSE}  # My User Event
        n102 = Create User Event(user event datatype=w263, error in=w261) -> (user event=w264:refnum<user-event>, error out=w260:errorcluster)
        n103 = property on="volume description" class="WebView2 Control (strict)"() -> ("Events"=w258:T11)  [unwired: 2 in, 2 out]
        n104 = register-events(error in=w260, w264, w258) -> (reference out=w262:refnum<event-registration>, error out=w259:errorcluster)  [unwired: 1 in]
        n105 = call <vilib>:"Add State(s) to Queue__jki_lib_state_machine.vi"("State(s) in (\"\")"=w267) -> ("States Out"=w266:string)  [unwired: 14 in]
      }
      frame "Events: Unregister" {
        n106 = Unregister For Events(event registration refnum=w270, error in=w269) -> (error out=w268:errorcluster)
        n107 = call <vilib>:"Add State(s) to Queue__jki_lib_state_machine.vi"("State(s) in (\"\")"=w273) -> ("States Out"=w272:string)  [unwired: 14 in]
      }
      frame "---------- UI ----------" {
        n108 = call <vilib>:"Add State(s) to Queue__jki_lib_state_machine.vi"("State(s) in (\"\")"=w278) -> ("States Out"=w277:string)  [unwired: 14 in]
      }
      frame "UI: Display Volumes" {
        n109 = Unbundle By Name(w287) -> ("vol_filter_map"=w289:map{i32, cluster{"name":string, "path":path}[]})
        n110 = local read "Folder"() -> (w288:i32)
        n111 = Look In Map(map=w289, key=w288) -> (value=w285:cluster{"name":string, "path":path}[])  [unwired: 1 in, 1 out]
        n112 = for {
          tunnel: w285 -> [w301] mode=indexing
          tunnel: [w300] -> w284 mode=indexing
          n113 = Unbundle By Name(w301) -> ("name"=w300:string)
        }
        n114 = local read "volumes"() -> (w280:i32)
        n115 = Bundle By Name(cluster=w287, "current_vol_array"=w285) -> (w286:T9)
        n116 = case shown="Default" w279 {
          tunnel: w284 -> [w295 w299]
          tunnel: w283 -> [w294 w298]
          tunnel: [w293 w297] -> w282
          tunnel: w280 -> [_ w296]
          frame "TRUE" {
            w292 = 0 ("Value (Signaling)")
            n117 = property on="volumes" class="LstBox (strict)"(error in=w294, "Item Names"=w295, "Val(Sgnl)"=w292, "Top Row"=w292) -> (error out=w293:errorcluster)  [unwired: 1 in, 1 out]
          }
          frame Default {
            n118 = property on="volumes" class="LstBox (strict)"(error in=w298, "Item Names"=w299, "Val(Sgnl)"=w296) -> (error out=w297:errorcluster)  [unwired: 1 in, 1 out]
          }
        }
        n119 = call <vilib>:"Add State(s) to Queue__jki_lib_state_machine.vi"("State(s) in (\"\")"=w291) -> ("States Out"=w290:string)  [unwired: 14 in]
      }
      frame "UI: Display Issues" {
        n120 = Unbundle By Name(w305) -> ("issues"=w304:T4[])
        n121 = Empty Array?(array=w304) -> (empty?=w303:bool)
        n122 = case shown="False" w303 {
          tunnel: w307 -> [w314 w326]
          tunnel: [w313 w326] -> w306
          tunnel: w304 -> [w312 _]
          tunnel: w302 -> [w311 _]
          frame False {
            n123 = for {
              tunnel: w312 -> [w325] mode=indexing
              tunnel: [w324] -> w315 mode=indexing
              n124 = Unbundle By Name(w325) -> ("sortable_name"=w324:string)
            }
            n125 = case shown="Default" w311 {
              tunnel: w315 -> [w319 w323]
              tunnel: w314 -> [w318 w322]
              tunnel: [w317 w321] -> w313
              frame Default {
                n126 = local read "issues"() -> (w316:i32)
                n127 = property on="issues" class="LstBox (strict)"(error in=w318, "Item Names"=w319, "Val(Sgnl)"=w316) -> (error out=w317:errorcluster)  [unwired: 1 in, 1 out]
              }
              frame "TRUE" {
                w320 = 0 ("Value (Signaling)")
                n128 = property on="issues" class="LstBox (strict)"(error in=w322, "Item Names"=w323, "Val(Sgnl)"=w320, "Top Row"=w320) -> (error out=w321:errorcluster)  [unwired: 1 in, 1 out]
              }
            }
          }
          frame True {
          }
        }
        n129 = call <vilib>:"Add State(s) to Queue__jki_lib_state_machine.vi"("State(s) in (\"\")"=w310) -> ("States Out"=w309:string)  [unwired: 14 in]
      }
      frame "UI: Ready" {
        n130 = call <vilib>:"Add State(s) to Queue__jki_lib_state_machine.vi"("State(s) in (\"\")"=w331) -> ("States Out"=w330:string)  [unwired: 14 in]
      }
      frame "UI: Populate Volume Info" {
        n131 = Unbundle By Name(w342) -> ("volume.date_last_updated"=w337:timestamp, "volume.volume"=w333:i32, "volume.start_year"=→"Start Year":i32, "volume.count_of_issues"=→"issue count":i32, "volume.sortable_name"=→"Sortable Title":string, "volume.name"=w332:string, "volume.description"=w338:string, "volume.volume type"=w335:T1, "volume.site_detail_url"=→"URL":string)
        n132 = Format Date/Time String(seconds (now)=w337) -> (date/time string=→"last updated":string)  [unwired: 2 in]
        n133 = local write "Volume"(w333) -> ()
        n134 = local write "Title"(w332) -> ()
        n135 = local write "volume type"(w335) -> ()
        n136 = property on="volume description" class="WebView2 Control (strict)"(error in=w345, "Document Source"=w338) -> (error out=w344:errorcluster)  [unwired: 1 in, 1 out]
        n137 = call <vilib>:"Add State(s) to Queue__jki_lib_state_machine.vi"("State(s) in (\"\")"=w347) -> ("States Out"=w346:string)  [unwired: 14 in]
      }
      frame "UI: Populate Issue Info" {
        n138 = Unbundle By Name(w373) -> ("issues"=w372:T4[])
        n139 = local read "issues"() -> (w371:i32)
        n140 = Index Array(array=w372, index=w371) -> (element=w370:T4)
        n141 = Unbundle By Name(w370) -> ("store_date"=→"Rel Date":timestamp, "cover_date"=w349:timestamp, "id"=→"Issue ID":i32, "name"=→"Issue Title":string, "issue_number"=→"Issue Number":string, "cover_url"=w366:string, "description"=w361:string, "characters"=w360:T5[], "concepts"=w358:T5[], "storyArcs"=w356:T5[], "teams"=w354:T5[], "creators"=w352:T7[])
        n142 = property on="issue description" class="WebView2 Control (strict)"(error in=w365, "Document Source"=w361) -> (error out=w364:errorcluster)  [unwired: 1 in, 1 out]
        n143 = property on="issue cover" class="WebView2 Control (strict)"(error in=w365, "URL"=w366) -> (error out=w363:errorcluster)  [unwired: 1 in, 1 out]
        n144 = local write "Cover Date"(w349) -> ()
        n145 = for {
          tunnel: w360 -> [w389] mode=indexing
          tunnel: [w388] -> w359 mode=indexing
          n146 = Unbundle By Name(w389) -> ("name"=w388:string)
        }
        "Characters" <- w359
        n147 = for {
          tunnel: w358 -> [w387] mode=indexing
          tunnel: [w386] -> w357 mode=indexing
          n148 = Unbundle By Name(w387) -> ("name"=w386:string)
        }
        "Concepts" <- w357
        n149 = for {
          tunnel: w356 -> [w385] mode=indexing
          tunnel: [w384] -> w355 mode=indexing
          n150 = Unbundle By Name(w385) -> ("name"=w384:string)
        }
        "StoryArcs" <- w355
        n151 = for {
          tunnel: w354 -> [w383] mode=indexing
          tunnel: [w382] -> w353 mode=indexing
          n152 = Unbundle By Name(w383) -> ("name"=w382:string)
        }
        "Teams" <- w353
        n153 = Merge Errors(w363, w364) -> (w362:errorcluster)
        n154 = for {
          tunnel: w352 -> [w381] mode=indexing
          tunnel: [w378] -> w351 mode=indexing
          tunnel: " - " ("string") -> [w377]
          n155 = Unbundle By Name(w381) -> ("name"=w380:string, "role"=w379:string)
          n156 = Concatenate Strings(w380, w377, w379) -> (w378:string)
        }
        "Creators" <- w351
        n157 = call <vilib>:"Add State(s) to Queue__jki_lib_state_machine.vi"("State(s) in (\"\")"=w376) -> ("States Out"=w375:string)  [unwired: 14 in]
      }
      frame "UI: Initialize" {
        # "Initialize the User Interface, here.\n(this is called automatically, by the Macro: Initialize)"
        n158 = call <vilib>:"Add State(s) to Queue__jki_lib_state_machine.vi"("State(s) in Front (\"\")"="Actions: Populate cv_vols\nActions: create volume filter map\nUI: Display Volumes >> TRUE\nActions: Load Volume\nUI: Ready" ("State(s) in Front (\"\")"), "State(s) in (\"\")"=w395) -> ("States Out"=w394:string)  [unwired: 13 in]
      }
      frame "UI: Uninitialize" {
        # "Cleanup the User Interface, here.\n(this is called automatically, by the Macro: Exit)"
        n159 = call <vilib>:"Add State(s) to Queue__jki_lib_state_machine.vi"("State(s) in (\"\")"=w400) -> ("States Out"=w399:string)  [unwired: 14 in]
      }
      frame "UI: Cursor Set" {
        # "Argument"
        # "Set and Unset Cursor Busy.\n(Usage: \"UI: Cursor Set >> Busy|Idle\")"
        n160 = case shown="\"Idle\", Default" w402 {
          tunnel: w404 -> [w409 w411]
          tunnel: [w408 w410] -> w403
          frame "Idle", Default {
            n161 = call <vilib>:"Unset Busy.vi"("error in (no error)"=w409) -> ("error out"=w408:errorcluster)  [unwired: 10 in]
          }
          frame "Busy" {
            n162 = call <vilib>:"Set Busy.vi"("error in (no error)"=w411) -> ("error out"=w410:errorcluster)  [unwired: 9 in, 1 out]
          }
        }
        n163 = call <vilib>:"Add State(s) to Queue__jki_lib_state_machine.vi"("State(s) in (\"\")"=w407) -> ("States Out"=w406:string)  [unwired: 14 in]
      }
      frame "UI: Front Panel State" {
        # "Argument"
        # "Set Front Panel Open or Closed\n(Usage: \"UI: Front Panel State >> Open|Close\")"
        n164 = Unbundle By Name(w415) -> ("Core.Current VI Reference"=w414:refnum<vi>)
        n165 = case shown="\"Open\", \"Standard\", Default" w413 {
          tunnel: w417 -> [w425 w440 w451 w464 w477]
          tunnel: [w427 w441 w453 w466 w479] -> w416
          tunnel: w414 -> [w426 w438 w452 w465 w478]
          frame "Open", "Standard", Default {
            w420 = T2."Standard" ("State")
            n166 = property class="VI"(reference=w426, error in=w425) -> (reference out=w423:refnum<vi>, error out=w424:errorcluster, "FP.State"=w422:T2)
            n167 = Not Equal?(x=w422, y=w420) -> (x != y?=w421:bool)
            n168 = case shown="False" w421 {
              tunnel: [w431 w433] -> w427
              tunnel: w424 -> [w430 w433]
              tunnel: w423 -> [w429 _]
              tunnel: w420 -> [w428 _]
              frame True {
                n169 = invoke class="VI" method="FP.Open"(reference=w429, error in=w430, "Activate"=TRUE, "State"=w428) -> (error out=w431:errorcluster)  [unwired: 1 in, 4 out]
              }
              frame False {
              }
            }
          }
          frame "Close", "Closed" {
            n170 = property class="VI"(reference=w438, error in=w440) -> (reference out=w437:refnum<vi>, error out=w439:errorcluster, "FP.State"=w435:T2)
            n171 = Not Equal?(x=w435, y=T2."Closed" ("Front Panel Window:State")) -> (x != y?=w434:bool)
            n172 = case shown="True" w434 {
              tunnel: [w442 w445] -> w441
              tunnel: w439 -> [w442 w444]
              tunnel: w437 -> [_ w443]
              frame False {
              }
              frame True {
                n173 = invoke class="VI" method="FP.Close"(reference=w443, error in=w444) -> (error out=w445:errorcluster)  [unwired: 1 in, 2 out]
              }
            }
          }
          frame "Hidden", "Hide" {
            w446 = T2."Hidden" ("State")
            n174 = property class="VI"(reference=w452, error in=w451) -> (reference out=w449:refnum<vi>, error out=w450:errorcluster, "FP.State"=w448:T2)
            n175 = Not Equal?(x=w448, y=w446) -> (x != y?=w447:bool)
            n176 = case shown="True" w447 {
              tunnel: [w457 w458] -> w453
              tunnel: w450 -> [w456 w458]
              tunnel: w449 -> [w455 _]
              tunnel: w446 -> [w454 _]
              frame True {
                n177 = invoke class="VI" method="FP.Open"(reference=w455, error in=w456, "State"=w454) -> (error out=w457:errorcluster)  [unwired: 2 in, 4 out]
              }
              frame False {
              }
            }
          }
          frame "Minimize", "Minimized" {
            w459 = T2."Minimized" ("State")
            n178 = property class="VI"(reference=w465, error in=w464) -> (reference out=w462:refnum<vi>, error out=w463:errorcluster, "FP.State"=w461:T2)
            n179 = Not Equal?(x=w461, y=w459) -> (x != y?=w460:bool)
            n180 = case shown="True" w460 {
              tunnel: [w470 w471] -> w466
              tunnel: w463 -> [w469 w471]
              tunnel: w462 -> [w468 _]
              tunnel: w459 -> [w467 _]
              frame True {
                n181 = invoke class="VI" method="FP.Open"(reference=w468, error in=w469, "State"=w467) -> (error out=w470:errorcluster)  [unwired: 2 in, 4 out]
              }
              frame False {
              }
            }
          }
          frame "Maximize", "Maximized" {
            w472 = T2."Maximized" ("State")
            n182 = property class="VI"(reference=w478, error in=w477) -> (reference out=w475:refnum<vi>, error out=w476:errorcluster, "FP.State"=w474:T2)
            n183 = Not Equal?(x=w474, y=w472) -> (x != y?=w473:bool)
            n184 = case shown="True" w473 {
              tunnel: [w483 w484] -> w479
              tunnel: w476 -> [w482 w484]
              tunnel: w475 -> [w481 _]
              tunnel: w472 -> [w480 _]
              frame True {
                n185 = invoke class="VI" method="FP.Open"(reference=w481, error in=w482, "State"=w480) -> (error out=w483:errorcluster)  [unwired: 2 in, 4 out]
              }
              frame False {
              }
            }
          }
        }
        n186 = call <vilib>:"Add State(s) to Queue__jki_lib_state_machine.vi"("State(s) in (\"\")"=w419) -> ("States Out"=w418:string)  [unwired: 14 in]
      }
      frame "---------- Macro ----------" {
        # "Do not put any code in this frame.\n(It is a separator no-op. You can make a copy of this frame to create a new Macro frame)"
        n187 = call <vilib>:"Add State(s) to Queue__jki_lib_state_machine.vi"("State(s) in (\"\")"=w489) -> ("States Out"=w488:string)  [unwired: 14 in]
      }
      frame "Macro: Initialize" {
        # "Initialization Macro\n(This is called once, when the VI starts)"
        n188 = call <vilib>:"Add State(s) to Queue__jki_lib_state_machine.vi"("State(s) in Front (\"\")"="Data: Initialize\nInitialize Core Data\nEvents: Register\nUI: Initialize\nUI: Front Panel State >> Open", "State(s) in (\"\")"=w495) -> ("States Out"=w494:string)  [unwired: 13 in]
      }
      frame "Macro: Exit" {
        # "Exit Macro\n(This is called once, when the VI exits)"
        n189 = Unbundle By Name(w503) -> ("Core.Close Panel on Exit?"=w498:bool)
        n190 = call <vilib>:"Conditional State String__jki_lib_state_machine.vi"("Do State(s)?"=w498, "State"="UI: Front Panel State >> Close") -> ("State Out"=w497:string)  [unwired: 7 in]
        n191 = call <vilib>:"Add State(s) to Queue__jki_lib_state_machine.vi"("State(s) in (\"\")"=w497, "State(s) at Back (\"\")"="UI: Uninitialize\nData: Cleanup\nEvents: Unregister\nExit") -> ("States Out"=w501:string)  [unwired: 13 in]
        n192 = call <vilib>:"Add State(s) to Queue__jki_lib_state_machine.vi"("State(s) in Front (\"\")"=w501, "State(s) in (\"\")"=w505) -> ("States Out"=w504:string)  [unwired: 13 in]
      }
      frame "---------- Actions ----------" {
        n193 = call <vilib>:"Add State(s) to Queue__jki_lib_state_machine.vi"("State(s) in (\"\")"=w510) -> ("States Out"=w509:string)  [unwired: 14 in]
      }
      frame "Actions: Delete Issue" {
        n194 = Unbundle By Name(w527) -> ("volume"=w530:T8, "issues"=w533:T4[])
        n195 = local read "issues"() -> (w521:i32)
        n196 = Unbundle By Name(w527) -> ("root paths.cv_volumes"=w519:path, "current_vol_array"=w526:cluster{"name":string, "path":path}[])
        n197 = local read "volumes"() -> (w525:i32)
        n198 = Delete From Array(array=w533, index=w521) -> (array with subset deleted=w529:T4[])  [unwired: 1 in, 1 out]
        n199 = Unbundle By Name(w530) -> ("count_of_issues"=w512:i32, "issue_ids"=w532:i32[])
        n200 = Index Array(array=w526, index=w525) -> (element=w524:cluster{"name":string, "path":path})
        n201 = Unbundle By Name(w524) -> ("path"=w523:path)
        n202 = Decrement(x=w512) -> (x-1=w511:i32)
        n203 = Delete From Array(array=w532, index=w521) -> (array with subset deleted=w528:i32[])  [unwired: 1 in, 1 out]
        n204 = Delete(path (use dialog)=w523, error in=w522) -> (error out=w518:errorcluster)  [unwired: 3 in, 2 out]
        n205 = Bundle By Name(cluster=w530, "count_of_issues"=w511, "issue_ids"=w528) -> (w514:T8)
        n206 = call "create.volume.filename.vi"("volume"=w514) -> ("json filename"=w520:string)  [unwired: 10 in]
        n207 = call <vilib>:"Flatten To JSON String.vi"("error in"=w518, "Variant"=w514) -> ("error out"=w517:errorcluster, "JSON String"=w516:string)  [unwired: 8 in]
        n208 = Build Path(base path=w519, name or relative path=w520) -> (appended path=w515:path)
        n209 = Bundle By Name(cluster=w527, "volume"=w514, "issues"=w529) -> (w531:T9)
        n210 = Write to Text File(file (use dialog)=w515, text=w516, error in=w517) -> (error out=w513:errorcluster)  [unwired: 1 in, 2 out]
        n211 = call <vilib>:"Add State(s) to Queue__jki_lib_state_machine.vi"("State(s) in (\"\")"=w536) -> ("States Out"=w535:string)  [unwired: 14 in]
      }
      frame "Actions: Change Volume" {
        n212 = Unbundle By Name(w551) -> ("volume"=w552:T8)
        n213 = Unbundle By Name(w551) -> ("root paths.cv_volumes"=w544:path, "current_vol_array"=w550:cluster{"name":string, "path":path}[])
        n214 = local read "volumes"() -> (w549:i32)
        n215 = Index Array(array=w550, index=w549) -> (element=w548:cluster{"name":string, "path":path})
        n216 = Unbundle By Name(w548) -> ("path"=w547:path)
        n217 = local read "Volume"() -> (w537:i32)
        n218 = Delete(path (use dialog)=w547, error in=w546) -> (error out=w543:errorcluster)  [unwired: 3 in, 2 out]
        n219 = Bundle By Name(cluster=w552, "volume"=w537) -> (w539:T8)
        n220 = call "create.volume.filename.vi"("volume"=w539) -> ("json filename"=w545:string)  [unwired: 10 in]
        n221 = call <vilib>:"Flatten To JSON String.vi"("error in"=w543, "Variant"=w539) -> ("error out"=w542:errorcluster, "JSON String"=w541:string)  [unwired: 8 in]
        n222 = Build Path(base path=w544, name or relative path=w545) -> (appended path=w540:path)
        n223 = Bundle By Name(cluster=w551, "volume"=w539) -> (w553:T9)
        n224 = Write to Text File(file (use dialog)=w540, text=w541, error in=w542) -> (error out=w538:errorcluster)  [unwired: 1 in, 2 out]
        n225 = call <vilib>:"Add State(s) to Queue__jki_lib_state_machine.vi"("State(s) in (\"\")"=w556) -> ("States Out"=w555:string)  [unwired: 14 in]
      }
      frame "Actions: Change Title" {
        n226 = Unbundle By Name(w576) -> ("volume"=w577:T8, "volume.start_year"=w558:i32)
        n227 = local read "Title"() -> (w562:string)
        n228 = Unbundle By Name(w576) -> ("root paths.cv_volumes"=w569:path, "current_vol_array"=w575:cluster{"name":string, "path":path}[])
        n229 = local read "volumes"() -> (w574:i32)
        n230 = call "MakeSortable.vi"("string in"=w562) -> ("string out"=w561:string)
        n231 = call "remove.invalid.chars.vi"("string in"=w561) -> ("string out"=w559:string)
        n232 = Index Array(array=w575, index=w574) -> (element=w573:cluster{"name":string, "path":path})
        n233 = Format Into String(format string="%s (%d)", w559, w558) -> (resulting string=w557:string)  [unwired: 2 in, 1 out]
        n234 = Unbundle By Name(w573) -> ("path"=w572:path)
        n235 = Delete(path (use dialog)=w572, error in=w571) -> (error out=w568:errorcluster)  [unwired: 3 in, 2 out]
        n236 = Bundle By Name(cluster=w577, "name"=w562, "sortable_name"=w557) -> (w564:T8)
        n237 = call "create.volume.filename.vi"("volume"=w564) -> ("json filename"=w570:string)  [unwired: 10 in]
        n238 = call <vilib>:"Flatten To JSON String.vi"("error in"=w568, "Variant"=w564) -> ("error out"=w567:errorcluster, "JSON String"=w566:string)  [unwired: 8 in]
        n239 = Build Path(base path=w569, name or relative path=w570) -> (appended path=w565:path)
        n240 = Bundle By Name(cluster=w576, "volume"=w564) -> (w578:T9)
        n241 = Write to Text File(file (use dialog)=w565, text=w566, error in=w567) -> (error out=w563:errorcluster)  [unwired: 1 in, 2 out]
        n242 = call <vilib>:"Add State(s) to Queue__jki_lib_state_machine.vi"("State(s) in (\"\")"=w581) -> ("States Out"=w580:string)  [unwired: 14 in]
      }
      frame "Actions: Change Dates to Rel Date" {
        n243 = Unbundle By Name(w586) -> ("issues"=w588:T4[], "root paths.cv_issues"=w587:path)
        n244 = for {
          tunnel: w588 -> [w602] mode=indexing
          tunnel: w587 -> [w598]
          tunnel: [w597] -> w585 mode=indexing
          shift-right: [w593] -> w583
          shift-left: w582 -> [w592]
          n245 = in-place {
            in-place-border: [w603] -> w600
            n246 = in-place-cluster #2(w602) -> ("store_date"=w604:timestamp, "id"=w603:i32)  [unwired: 1 out]
            n247 = in-place-cluster #2("cover_date"=w604, "store_date"=w604, "id"=w603) -> (w597:T4)
          }
          n248 = Format Into String(format string="%d.json", w600) -> (resulting string=w599:string)  [unwired: 2 in, 1 out]
          n249 = Build Path(base path=w598, name or relative path=w599) -> (appended path=w596:path)
          n250 = call <vilib>:"Flatten To JSON String.vi"("error in"=w592, "Variant"=w597) -> ("error out"=w594:errorcluster, "JSON String"=w595:string)  [unwired: 8 in]
          n251 = Write to Text File(file (use dialog)=w596, text=w595, error in=w594) -> (error out=w593:errorcluster)  [unwired: 1 in, 2 out]
        }
        n252 = Bundle By Name(cluster=w586, "issues"=w585) -> (w584:T9)
        n253 = call <vilib>:"Add State(s) to Queue__jki_lib_state_machine.vi"("State(s) in (\"\")"=w591) -> ("States Out"=w590:string)  [unwired: 14 in]
      }
      frame "Actions: Draw Issues" {
        n254 = Unbundle By Name(w613) -> ("volume.volume type"=w605:T1, "volume.sortable_name"=w606:string, "issues"=w612:T4[])
        n255 = for {
          tunnel: w612 -> [w619] mode=indexing
          tunnel: [w618] -> w610 mode=indexing
          tunnel: [w617] -> w609 mode=indexing
          n256 = Unbundle By Name(w619) -> ("issue_number"=w617:string, "cover_date"=w618:timestamp)
        }
        n257 = control-ref of="issue chart"() -> (w611:refnum<vi>)
        n258 = call "plot.issues.vi"("volume.volume type"=w605, "volume_name"=w606, "error in (no error)"=w608, "cover_dates"=w610, "issue_numbers"=w609, "picture ref"=w611) -> ("error out"=w607:errorcluster)  [unwired: 4 in, 1 out]
        n259 = call <vilib>:"Add State(s) to Queue__jki_lib_state_machine.vi"("State(s) in (\"\")"=w616) -> ("States Out"=w615:string)  [unwired: 14 in]
      }
      frame "Actions: Clean Cover Dates" {
        n260 = Unbundle By Name(w625) -> ("issues"=w627:T4[], "dup issues"=w626:i32[], "root paths.cv_issues"=w622:path)
        n261 = call "interpolate.issue.dates.vi"("dup issues"=w626, "issues"=w627) -> ("issues out"=w623:T4[])  [unwired: 9 in]
        n262 = for {
          tunnel: w626 -> [w641] mode=indexing
          tunnel: w623 -> [w642]
          tunnel: w622 -> [w636]
          shift-right: [w631] -> w620
          shift-left: w621 -> [w632]
          n263 = Index Array(array=w642, index=w641) -> (element=w640:T4)
          n264 = Unbundle By Name(w640) -> ("id"=w639:i32)
          n265 = call <vilib>:"Flatten To JSON String.vi"("error in"=w632, "Variant"=w640) -> ("error out"=w633:errorcluster, "JSON String"=w634:string)  [unwired: 8 in]
          n266 = Format Into String(format string="%d.json", w639) -> (resulting string=w637:string)  [unwired: 2 in, 1 out]
          n267 = Build Path(base path=w636, name or relative path=w637) -> (appended path=w635:path)
          n268 = Write to Text File(file (use dialog)=w635, text=w634, error in=w633) -> (error out=w631:errorcluster)  [unwired: 1 in, 2 out]
        }
        n269 = Bundle By Name(cluster=w625, "issues"=w623) -> (w624:T9)
        n270 = call <vilib>:"Add State(s) to Queue__jki_lib_state_machine.vi"("State(s) in (\"\")"=w630) -> ("States Out"=w629:string)  [unwired: 14 in]
      }
      frame "Actions: Delete Volume" {
        n271 = Unbundle By Name(w652) -> ("root paths.cv_issues"=w648:path, "volume.issue_ids"=w649:i32[], "current_vol_array"=w651:cluster{"name":string, "path":path}[])
        n272 = local read "volumes"() -> (w650:i32)
        n273 = Index Array(array=w651, index=w650) -> (element=w647:cluster{"name":string, "path":path})
        n274 = Unbundle By Name(w647) -> ("path"=w646:path)
        n275 = Delete(path (use dialog)=w646, error in=w645) -> (error out=w644:errorcluster)  [unwired: 3 in, 2 out]
        n276 = for {
          tunnel: w649 -> [w661] mode=indexing
          tunnel: w648 -> [w659]
          shift-right: [w656] -> w643
          shift-left: w644 -> [w657]
          n277 = Format Into String(format string="%d.json", w661) -> (resulting string=w660:string)  [unwired: 2 in, 1 out]
          n278 = Build Path(base path=w659, name or relative path=w660) -> (appended path=w658:path)
          n279 = Delete(path (use dialog)=w658, error in=w657) -> (error out=w656:errorcluster)  [unwired: 3 in, 2 out]
        }
        n280 = call <vilib>:"Add State(s) to Queue__jki_lib_state_machine.vi"("State(s) in (\"\")"=w655) -> ("States Out"=w654:string)  [unwired: 14 in]
      }
      frame "Actions: Sort Volume" {
        n281 = Unbundle By Name(w670) -> ("current_vol_array"=w669:cluster{"name":string, "path":path}[], "root paths.cv_issues"=w668:path)
        n282 = local read "volumes"() -> (w665:i32)
        n283 = Index Array(array=w669, index=w665) -> (element=w664:cluster{"name":string, "path":path})
        n284 = Unbundle By Name(w664) -> ("path"=w663:path)
        n285 = call "sort.volume.issues.vi"("error in"=w671, "issues path"=w668, "volume path"=w663) -> ("error out"=w667:errorcluster)  [unwired: 8 in]
        n286 = property on="volumes" class="LstBox (strict)"(error in=w667, "Val(Sgnl)"=w665) -> (error out=w666:errorcluster)  [unwired: 1 in, 1 out]
        n287 = call <vilib>:"Add State(s) to Queue__jki_lib_state_machine.vi"("State(s) in (\"\")"=w674) -> ("States Out"=w673:string)  [unwired: 14 in]
      }
      frame "Actions: Update Volume Type" {
        n288 = Unbundle By Name(w677) -> ("current_vol_array"=w688:cluster{"name":string, "path":path}[])
        n289 = local read "volume type"() -> (w676:T1)
        n290 = local read "volumes"() -> (w687:i32)
        n291 = Index Array(array=w688, index=w687) -> (element=w686:cluster{"name":string, "path":path})
        n292 = Unbundle By Name(w686) -> ("path"=w678:path)
        n293 = Bundle By Name(cluster=w677, "volume.volume type"=w676) -> (w675:T9)
        n294 = call "open.local.volume.file.vi"("error in (no error)"=w685, "volume json"=w678) -> ("error out"=w682:errorcluster, "volume"=w684:T8)  [unwired: 8 in]
        n295 = Bundle By Name(cluster=w684, "volume type"=w676) -> (w681:T8)
        n296 = call <vilib>:"Flatten To JSON String.vi"("error in"=w682, "Variant"=w681) -> ("error out"=w680:errorcluster, "JSON String"=w683:string)  [unwired: 8 in]
        n297 = Write to Text File(file (use dialog)=w678, text=w683, error in=w680) -> (error out=w679:errorcluster)  [unwired: 1 in, 2 out]
        n298 = call <vilib>:"Add State(s) to Queue__jki_lib_state_machine.vi"("State(s) in (\"\")"=w691) -> ("States Out"=w690:string)  [unwired: 14 in]
      }
      frame "Actions: Move Issue Up" {
        n299 = Unbundle By Name(w710) -> ("current_vol_array"=w698:cluster{"name":string, "path":path}[], "volume"=w704:T8, "volume.issue_ids"=w709:i32[])
        n300 = local read "volumes"() -> (w695:i32)
        n301 = local read "issues"() -> (w705:i32)
        n302 = Index Array(array=w698, index=w695) -> (element=w697:cluster{"name":string, "path":path})
        n303 = Delete From Array(array=w709, length=1, index=w705) -> (deleted portion=w706:i32[], array with subset deleted=w707:i32[])
        n304 = Decrement(x=w705) -> (x-1=w692:i32)
        n305 = Unbundle By Name(w697) -> ("path"=w696:path)
        n306 = Insert Into Array(array=w707, index=w692, new element=w706) -> (w703:i32[])
        n307 = local write "issues"(w692) -> ()
        n308 = Bundle By Name(cluster=w704, "issue_ids"=w703) -> (w702:T8)
        n309 = call <vilib>:"Flatten To JSON String.vi"("error in"=w700, "Variant"=w702) -> ("error out"=w701:errorcluster, "JSON String"=w699:string)  [unwired: 8 in]
        n310 = Write to Text File(file (use dialog)=w696, text=w699, error in=w701) -> (error out=w694:errorcluster)  [unwired: 1 in, 2 out]
        n311 = property on="volumes" class="LstBox (strict)"(error in=w694, "Val(Sgnl)"=w695) -> (error out=w693:errorcluster)  [unwired: 1 in, 1 out]
        n312 = call <vilib>:"Add State(s) to Queue__jki_lib_state_machine.vi"("State(s) in (\"\")"=w713) -> ("States Out"=w712:string)  [unwired: 14 in]
      }
      frame "Actions: Move Issue Top" {
        w715 = 0 ("issues")
        n313 = Unbundle By Name(w734) -> ("current_vol_array"=w722:cluster{"name":string, "path":path}[], "volume"=w728:T8, "volume.issue_ids"=w733:i32[])
        n314 = local read "volumes"() -> (w719:i32)
        n315 = local read "issues"() -> (w729:i32)
        n316 = Index Array(array=w722, index=w719) -> (element=w721:cluster{"name":string, "path":path})
        n317 = Delete From Array(array=w733, length=1, index=w729) -> (deleted portion=w730:i32[], array with subset deleted=w731:i32[])
        n318 = Unbundle By Name(w721) -> ("path"=w720:path)
        n319 = Insert Into Array(array=w731, index=0, new element=w730) -> (w727:i32[])
        n320 = Bundle By Name(cluster=w728, "issue_ids"=w727) -> (w726:T8)
        n321 = call <vilib>:"Flatten To JSON String.vi"("error in"=w724, "Variant"=w726) -> ("error out"=w725:errorcluster, "JSON String"=w723:string)  [unwired: 8 in]
        n322 = Write to Text File(file (use dialog)=w720, text=w723, error in=w725) -> (error out=w718:errorcluster)  [unwired: 1 in, 2 out]
        n323 = property on="volumes" class="LstBox (strict)"(error in=w718, "Val(Sgnl)"=w719) -> (error out=w717:errorcluster)  [unwired: 1 in, 1 out]
        n324 = property on="issues" class="LstBox (strict)"(error in=w717, "Value"=w715, "Top Row"=w715) -> (error out=w716:errorcluster)  [unwired: 1 in, 1 out]
        n325 = call <vilib>:"Add State(s) to Queue__jki_lib_state_machine.vi"("State(s) in (\"\")"=w737) -> ("States Out"=w736:string)  [unwired: 14 in]
      }
      frame "Actions: Move Issue Down" {
        n326 = Unbundle By Name(w756) -> ("current_vol_array"=w744:cluster{"name":string, "path":path}[], "volume"=w750:T8, "volume.issue_ids"=w755:i32[])
        n327 = local read "volumes"() -> (w741:i32)
        n328 = local read "issues"() -> (w751:i32)
        n329 = Index Array(array=w744, index=w741) -> (element=w743:cluster{"name":string, "path":path})
        n330 = Delete From Array(array=w755, length=1, index=w751) -> (deleted portion=w752:i32[], array with subset deleted=w753:i32[])
        n331 = Increment(x=w751) -> (x+1=w738:i32)
        n332 = Unbundle By Name(w743) -> ("path"=w742:path)
        n333 = Insert Into Array(array=w753, index=w738, new element=w752) -> (w749:i32[])
        n334 = local write "issues"(w738) -> ()
        n335 = Bundle By Name(cluster=w750, "issue_ids"=w749) -> (w748:T8)
        n336 = call <vilib>:"Flatten To JSON String.vi"("error in"=w746, "Variant"=w748) -> ("error out"=w747:errorcluster, "JSON String"=w745:string)  [unwired: 8 in]
        n337 = Write to Text File(file (use dialog)=w742, text=w745, error in=w747) -> (error out=w740:errorcluster)  [unwired: 1 in, 2 out]
        n338 = property on="volumes" class="LstBox (strict)"(error in=w740, "Val(Sgnl)"=w741) -> (error out=w739:errorcluster)  [unwired: 1 in, 1 out]
        n339 = call <vilib>:"Add State(s) to Queue__jki_lib_state_machine.vi"("State(s) in (\"\")"=w759) -> ("States Out"=w758:string)  [unwired: 14 in]
      }
      frame "Actions: Load Volume" {
        w765 = T8 {"id"=0, "name"="", "sortable_name"="", "aliases"=[], "description"="", "site_detail_url"="", "count_of_issues"=0, "start_year"=0, "publisher_id"=0, "issue_ids"=[], "date_last_updated"=timestamp(0 s since 1904-01-01), "volume"=0, "cv_id"="", "volume type"=enum."One Shot"} ("volume")
        n340 = Unbundle By Name(w762) -> ("current_vol_array"=w774:cluster{"name":string, "path":path}[])
        n341 = local read "volumes"() -> (w773:i32)
        n342 = Index Array(array=w774, index=w773) -> (element=w772:cluster{"name":string, "path":path})
        n343 = Unbundle By Name(w772) -> ("path"=w771:path)
        n344 = Read from Text File(file (use dialog)=w771, error in=w770) -> (text=w768:string, error out=w769:errorcluster)  [unwired: 2 in, 2 out]
        n345 = call <vilib>:"Unflatten From JSON String.vi"("Type and Defaults"=w765, "error in"=w769, "JSON String"=w768) -> ("error out"=w767:errorcluster, "Variant"=w766:variant)  [unwired: 7 in]
        n346 = Variant To Data(error in=w767, type=w765, Variant=w766) -> (data=w760:T8, error out=w764:errorcluster)
        n347 = Bundle By Name(cluster=w762, "volume"=w760) -> (w761:T9)
        n348 = call <vilib>:"Add State(s) to Queue__jki_lib_state_machine.vi"("State(s) in (\"\")"=w776) -> ("States Out"=w775:string)  [unwired: 14 in]
      }
      frame "Actions: Load Issues" {
        n349 = Unbundle By Name(w784) -> ("root paths.cv_issues"=w780:path, "volume.issue_ids"=w787:i32[])
        n350 = for {
          tunnel: w787 -> [w801] mode=indexing
          tunnel: "%d.json" -> [w802]
          tunnel: w780 -> [w799]
          shift-right: [w793] -> w781
          shift-left: w785 -> [w797]
          tunnel: [w792] -> w783 mode=indexing if=w790
          tunnel: [w791] -> w779 mode=indexing if=w790
          n351 = Format Into String(format string=w802, w801) -> (resulting string=w800:string)  [unwired: 2 in, 1 out]
          n352 = Build Path(base path=w799, name or relative path=w800) -> (appended path=w798:path)
          n353 = call <vilib>:"Check if File or Folder Exists.vi"("error in (no error)"=w797, "path"=w798) -> ("error out"=w794:errorcluster, "file or folder exists?"=w796:bool, "dup path"=w795:path)  [unwired: 7 in]
          n354 = case shown="True" w796 {
            selector: w796 -> [w803 w806]
            tunnel: w795 -> [_ w815]
            tunnel: w794 -> [w804 w814]
            tunnel: [_ w808] -> w792
            tunnel: [w804 w807] -> w793
            tunnel: [w803 w806] -> w790
            tunnel: [_ w805] -> w791
            frame False {
            }
            frame True {
              w809 = T4 {"cover_date"=timestamp(0 s since 1904-01-01), "id"=0, "cv_id"="", "name"="", "sortable_name"="", "issue_number"="", "deck"="", "description"="", "volume"={"id"=0, "name"=""}, "store_date"=timestamp(0 s since 1904-01-01), "date_last_updated"=timestamp(0 s since 1904-01-01), "site_detail_url"="", "cover_url"="", "associated_images"=[], "characters"=[], "concepts"=[], "creators"=[], "storyArcs"=[], "teams"=[]} ("issue")
              n355 = Read from Text File(file (use dialog)=w815, error in=w814) -> (text=w812:string, error out=w813:errorcluster)  [unwired: 2 in, 2 out]
              n356 = call <vilib>:"Unflatten From JSON String.vi"("Type and Defaults"=w809, "error in"=w813, "JSON String"=w812) -> ("error out"=w811:errorcluster, "Variant"=w810:variant)  [unwired: 7 in]
              n357 = Variant To Data(error in=w811, type=w809, Variant=w810) -> (data=w808:T4, error out=w807:errorcluster)
              n358 = Unbundle By Name(w808) -> ("cover_date"=w805:timestamp)
            }
          }
        }
        n359 = call-poly <userlib>:"Remove Duplicates from 1D Array__ogtk.vi"("Input Array"=w779) -> ("indices of removed elements"=w777:i32[])  [unwired: 1 out]
        "dup issues" <- w777
        n360 = Empty Array?(array=w777) -> (empty?=→"Unique Dates":bool)
        n361 = Bundle By Name(cluster=w784, "dup issues"=w777, "issues"=w783) -> (w782:T9)
      }
      frame "Actions: Populate cv_vols" {
        n362 = Unbundle By Name(w817) -> ("root paths.cv_volumes"=w816:path)
        n363 = call <vilib>:"Recursive File List.vi"("pattern"="*.json", "error in (no error)"=w819, "Folder Path"=w816) -> ("error out"=w820:errorcluster, "All Files in Dir"=w822:path[])  [unwired: 4 in, 3 out]
        n364 = Bundle By Name(cluster=w817, "cv_vols"=w822) -> (w821:T9)
        n365 = call <vilib>:"Add State(s) to Queue__jki_lib_state_machine.vi"("State(s) in (\"\")"=w825) -> ("States Out"=w824:string)  [unwired: 14 in]
      }
      frame "Actions: create volume filter map" {
        n366 = property on="Folder" class="LstBox (strict)"(error in=w827) -> (error out=w828:errorcluster, "Item Names"=w835:string[])  [unwired: 1 in, 1 out]
        n367 = Unbundle By Name(w831) -> ("cv_vols"=w833:path[])
        n368 = To Lower Case(string=w835) -> (all lower case string=w834:string[])
        n369 = for {
          tunnel: w834 -> [w851]
          tunnel: w833 -> [w850] mode=indexing
          shift-right: [w845] -> w830
          shift-left: map{i32, cluster{"name":string, "path":path}[]} {} ("map") -> [w847]
          n370 = Strip Path(path=w850) -> (name=w853:string)  [unwired: 1 out]
          n371 = call-poly <userlib>:"Strip Path Extension__ogtk.vi"("path"=w853) -> ("root"=w842:string)  [unwired: 1 out]
          n372 = String Subset(string=w842, length (rest)=1 ("length (rest)")) -> (substring=w838:string)  [unwired: 1 in]
          n373 = Equal?(x=w838, y="'" ("x")) -> (x = y?=w840:bool)
          n374 = Select(t="n" ("x"), s=w840, f=w838) -> (s? t:f=w837:string)
          n375 = Decimal String To Number(string=w837) -> (offset past number=w852:i32)  [unwired: 2 in, 1 out]
          n376 = case shown="0" w852 {
            tunnel: w837 -> [w866 _]
            tunnel: w851 -> [w867 _]
            tunnel: [w865 0 ("index of element")] -> w846
            frame 0 {
              n377 = Search 1D Array(1D array=w867, element=w866) -> (index of element=w865:i32)  [unwired: 1 in]
            }
            frame Default {
            }
          }
          n378 = Bundle("root"=w842, "cv_vols"=w850) -> (w849:cluster{"root":string, "cv_vols":path})  [unwired: 1 in]
          n379 = Look In Map(map=w847, key=w846) -> (key not found?=w848:bool, value=w844:cluster{"name":string, "path":path}[])  [unwired: 1 in]
          n380 = case shown="False" w848 {
            tunnel: w849 -> [w857 w862]
            tunnel: w847 -> [w856 w864]
            tunnel: w846 -> [w854 w863]
            tunnel: [w855 w860] -> w845
            tunnel: w844 -> [w858 _]
            frame False {
              n381 = Build Array (concatenate)(w858, w857) -> (w859:cluster{"root":string, "cv_vols":path}[])
              n382 = Insert Into Map(map in=w856, key=w854, value=w859) -> (map out=w855:map{i32, cluster{"name":string, "path":path}[]})  [unwired: 2 out]
            }
            frame True {
              n383 = Build Array(w862) -> (w861:cluster{"root":string, "cv_vols":path}[])
              n384 = Insert Into Map(map in=w864, key=w863, value=w861) -> (map out=w860:map{i32, cluster{"name":string, "path":path}[]})  [unwired: 2 out]
            }
          }
        }
        n385 = Bundle By Name(cluster=w831, "vol_filter_map"=w830) -> (w829:T9)
      }
    }
  }
